vi "PictureControlIMAQReplacement.vi"() -> ()   [LabVIEW 2019]
uses:
  <vilib>/Utility/miscctls.llb/LVPoint32TypeDef.ctl
  <vilib>/Utility/miscctls.llb/LVPointTypeDef.ctl
  <vilib>/Utility/miscctls.llb/LVBoundsTypeDef.ctl
  <vilib>/Utility/error.llb/whitespace.ctl
  <userlib>/_OpenG.lib/array/array.llb/Reverse 2D Array (SGL)__ogtk.vi
  <vilib>/picture/picture.llb/Draw True-Color Pixmap.vi
  <vilib>/Dataflowg/G-Image/G-Image/Image Processing/Polymorphic VIs/Resize Image (Scale).vi
  Classes/Render/BigMAQ/BigMAQ.lvclass
  <vilib>/Dataflowg/G-Image/G-Image/G-Image.lvlib
panel:
  out "size(s) 3":i32
  out "size(s) 2":i32
  out "new picture":picture
  out "Array":picture[](array[picture])
  in  "Basename":string
  out "error out":errorcluster
  in  "error in (no error)":errorcluster
  out "Notes LUT":variant
  in  "Path":path
  out "NewVal":T1(ring)
  in  "Selection":T1(radio)
  out "Button":u16
  out "Draw Area Size":T2
  out "Origin":T3
  out "x-y":T4
  out "2D Picture":picture
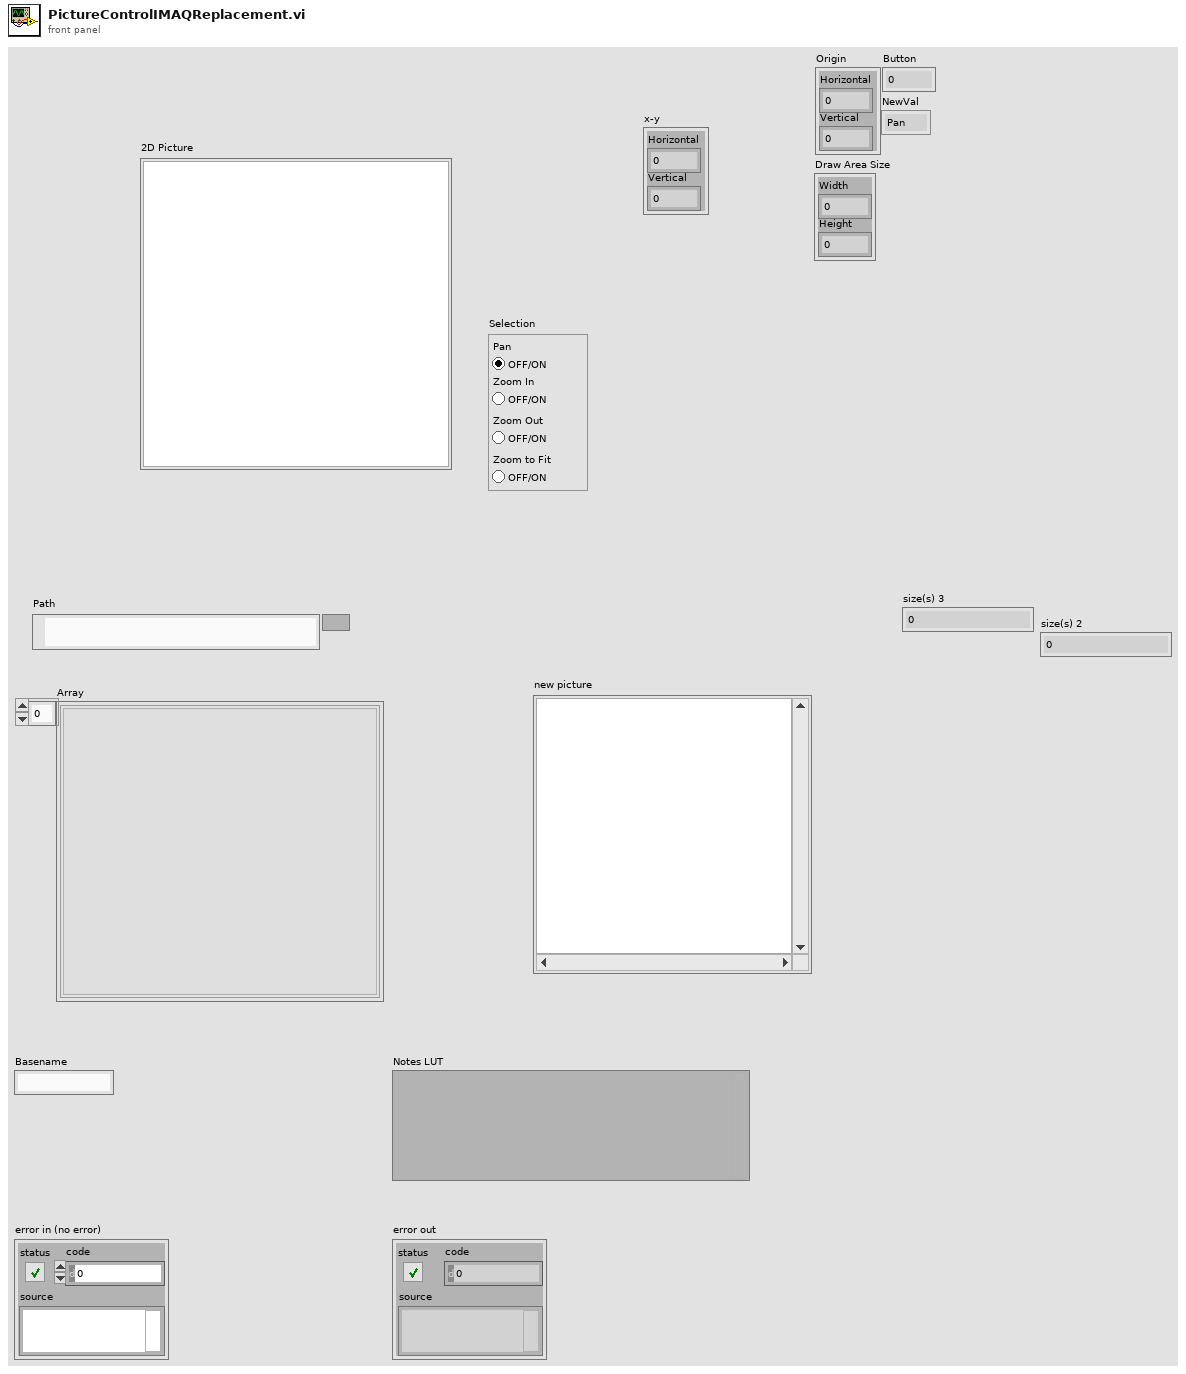
[diagram p1: front panel]
types:
  T1 = enum32{"Pan", "Zoom In", "Zoom Out", "Zoom to Fit"}
  T2 = typedef "LVBoundsTypeDef.ctl" = cluster{"Width":u32, "Height":u32}
  T3 = typedef "LVPointTypeDef.ctl" = cluster{"Horizontal":i16, "Vertical":i16}
  T4 = typedef "LVPoint32TypeDef.ctl" = cluster{"Horizontal":i32, "Vertical":i32}
  T5 = enum32{"Invalid", "Standard", "Closed", "Hidden", "Minimized", "Maximized"}
  T6 = enum32{"invalid app kind", "Development System", "Run Time System", "Student Edition", "Embedded LabVIEW", "Evaluation", "Custom"}
  T7 = enum16{"big-endian, network order", "native, host order", "little-endian"}
  T8 = cluster{"Core":cluster{"Current VI Reference":refnum<vi>, "Close Panel on Exit?":bool}, "Binary":string, "wfmSize":i32, "noteSize":i32, "nDim":i32[], "wData":sgl[], "Shaped wData":sgl[][][], "Notes":string, "Images":refnum<data-value>[]}
  T9 = cluster{"Current VI Reference":refnum<vi>, "Close Panel on Exit?":bool}
  T10 = typedef "whitespace.ctl" = u16
  T11 = typedef "imagedata.ctl" = cluster{"image type":i32, "image depth":i32, "image":u8[], "mask":u8[], "colors":u32[], "Rectangle":cluster{"left":i16, "top":i16, "right":i16, "bottom":i16}}
  T12 = cluster{"Core":cluster{"Current VI Reference":refnum<vi>, "Close Panel on Exit?":bool}, "MD Coords":T4, "MU Coords":T4, "MD":bool, "MD Origin":T4, "Selection":enum32{"Pan", "Zoom In", "Zoom Out", "Zoom to Fit"}}
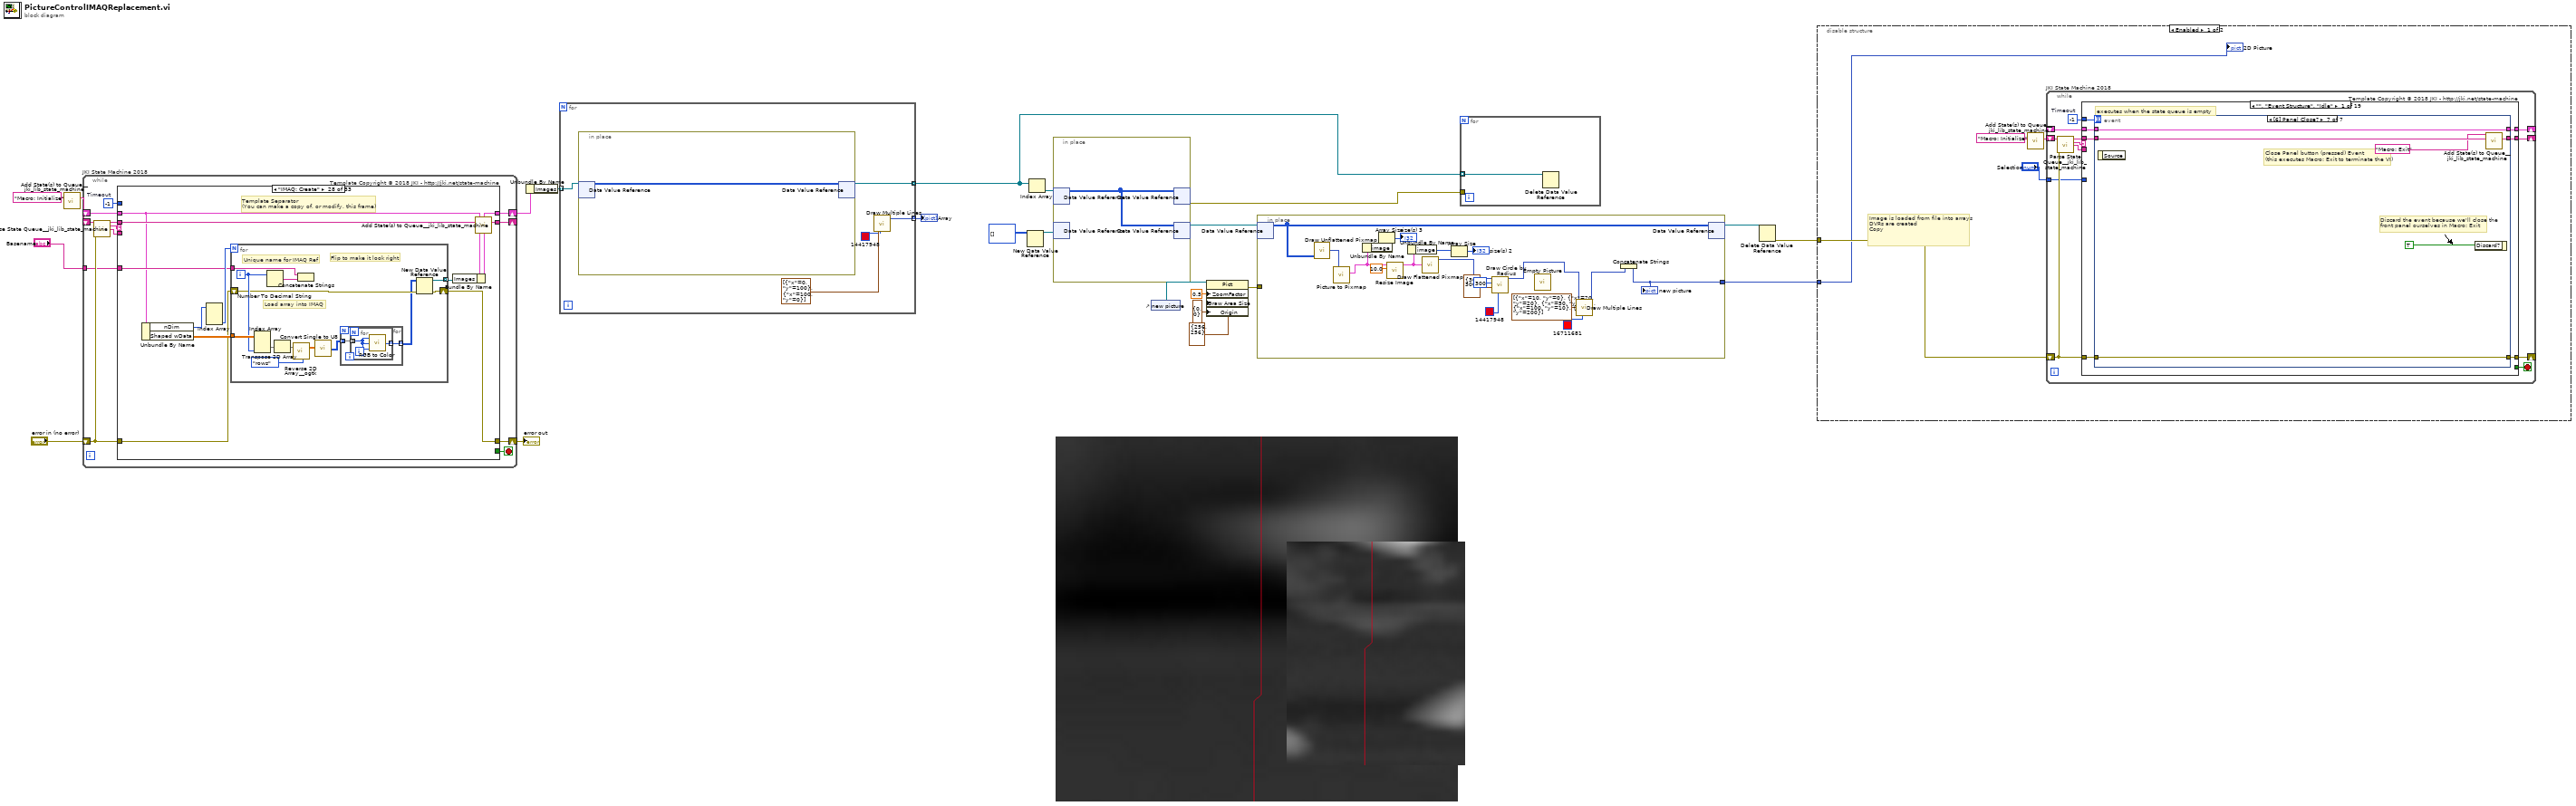
[diagram p0: block diagram]
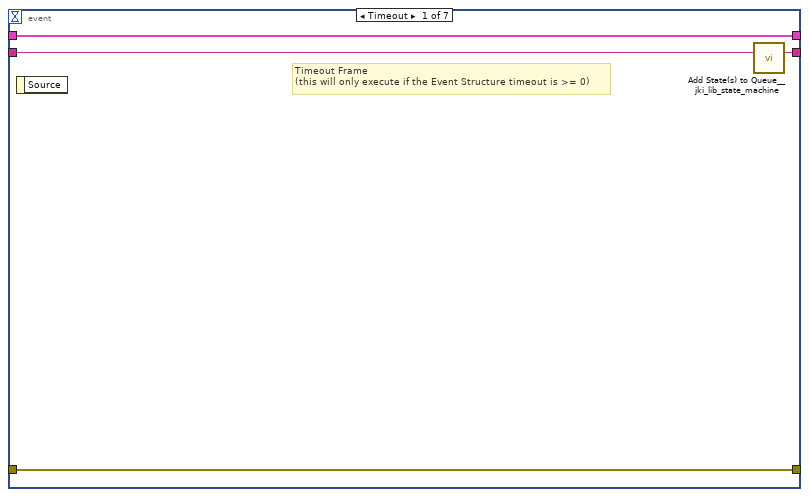
[diagram p2: hidden frame]
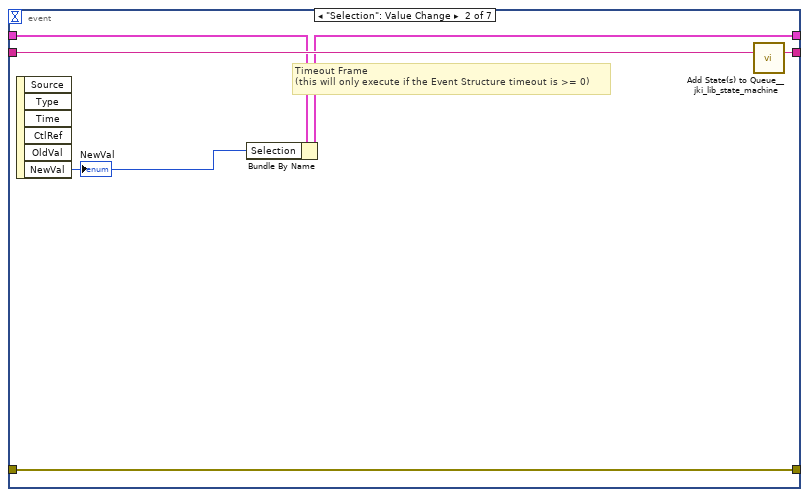
[diagram p3: hidden frame]
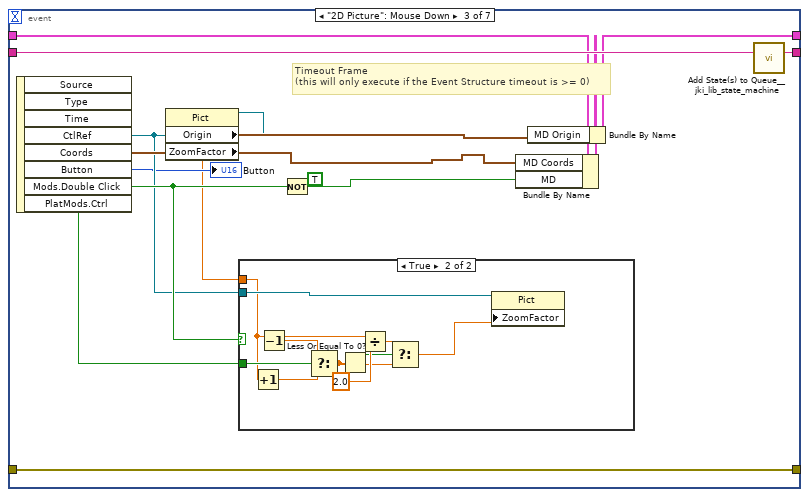
[diagram p4: hidden frame]
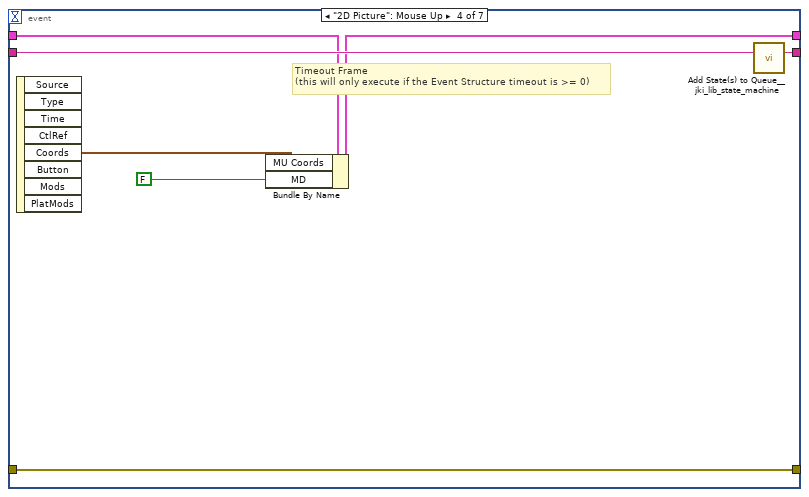
[diagram p6: hidden frame]
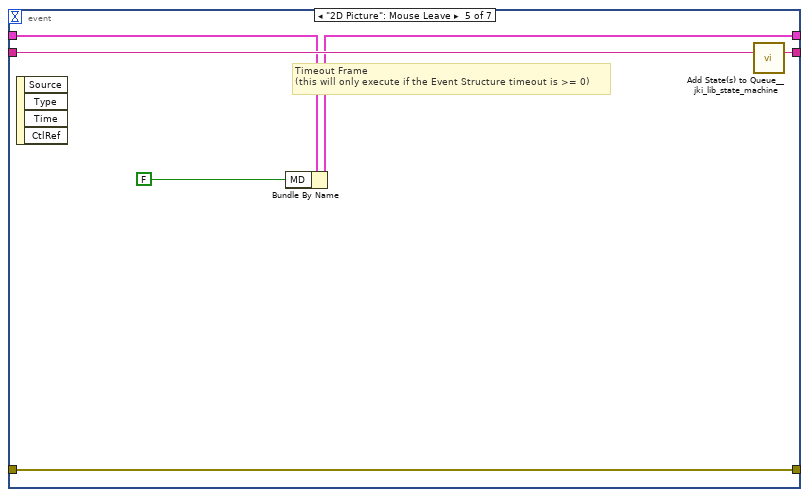
[diagram p7: hidden frame]
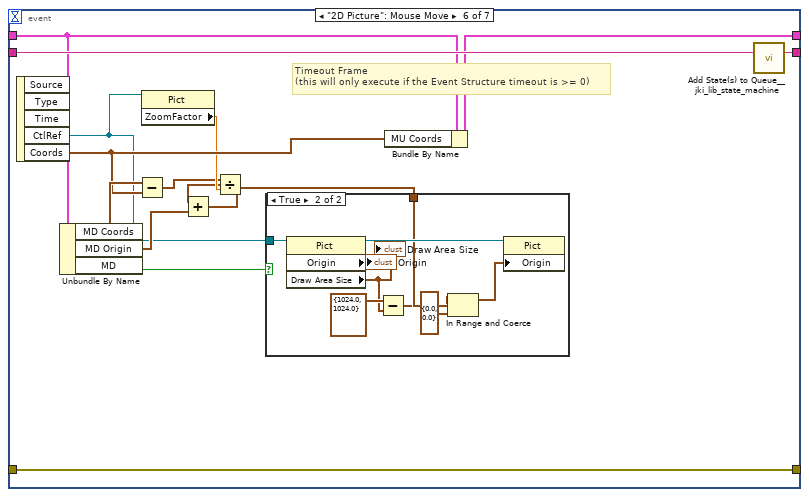
[diagram p8: hidden frame]
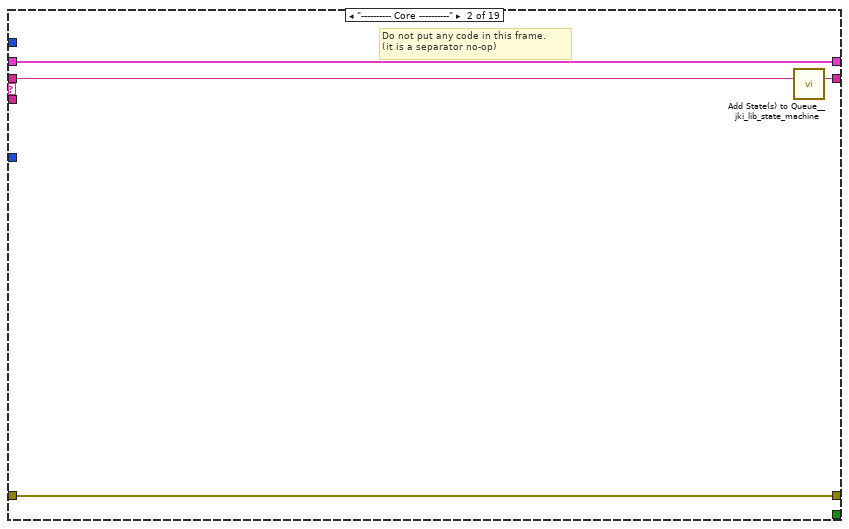
[diagram p10: hidden frame]
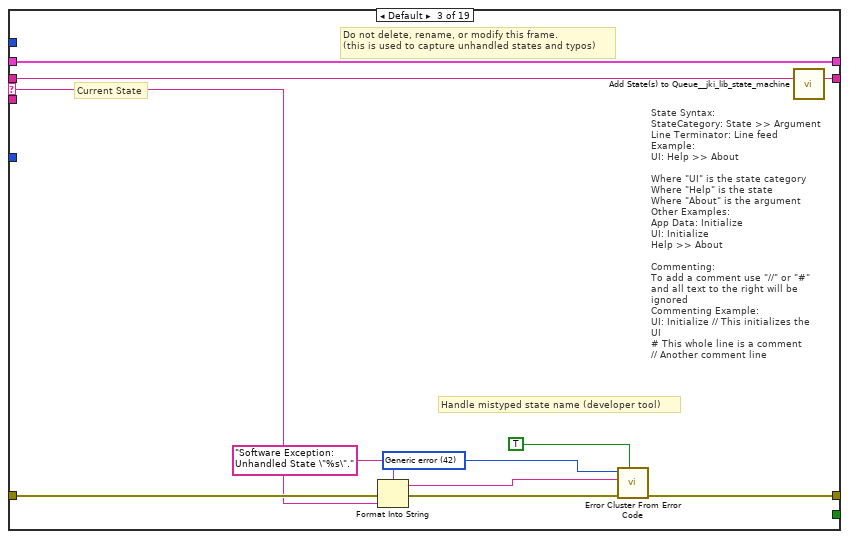
[diagram p11: hidden frame]
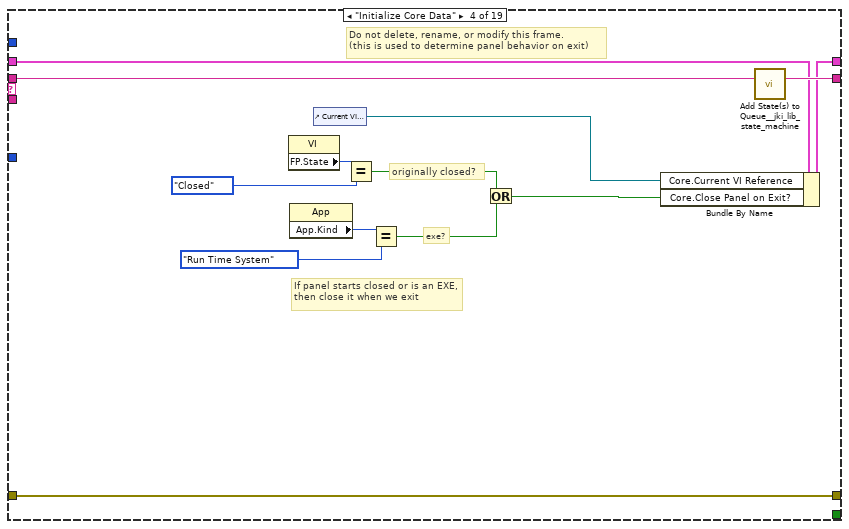
[diagram p12: hidden frame]
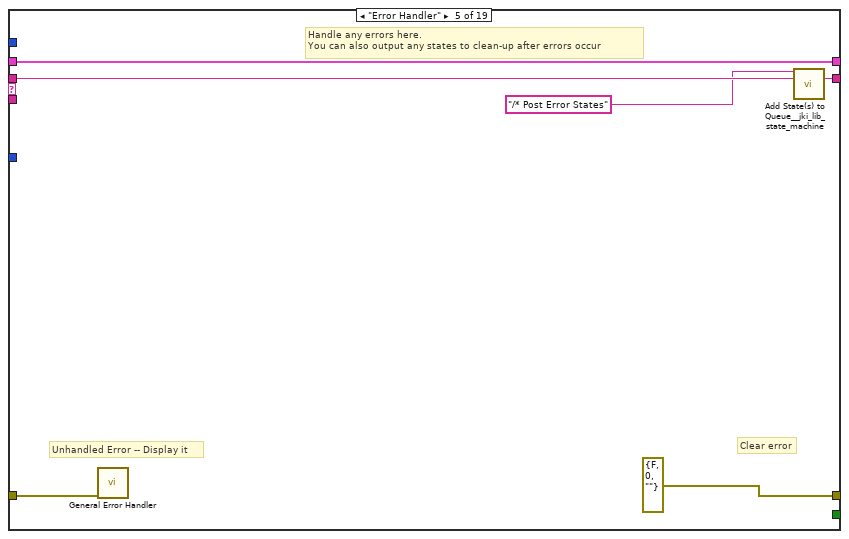
[diagram p13: hidden frame]
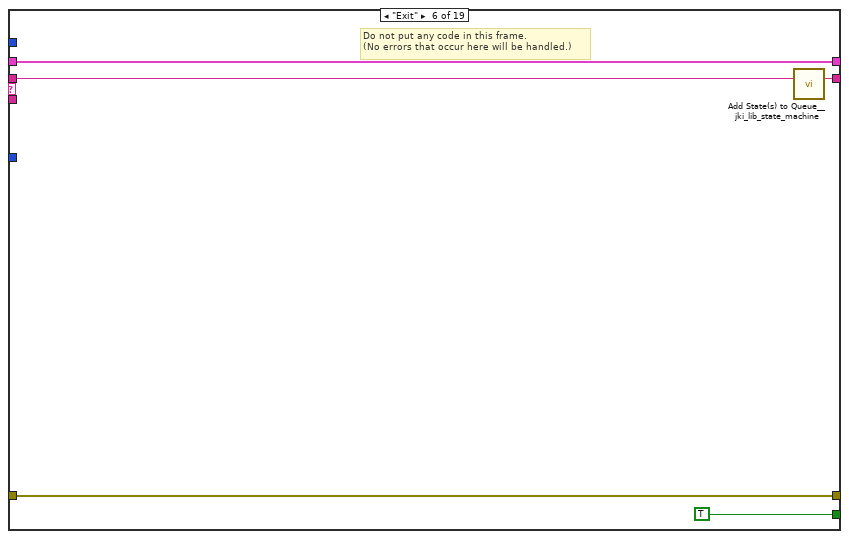
[diagram p14: hidden frame]
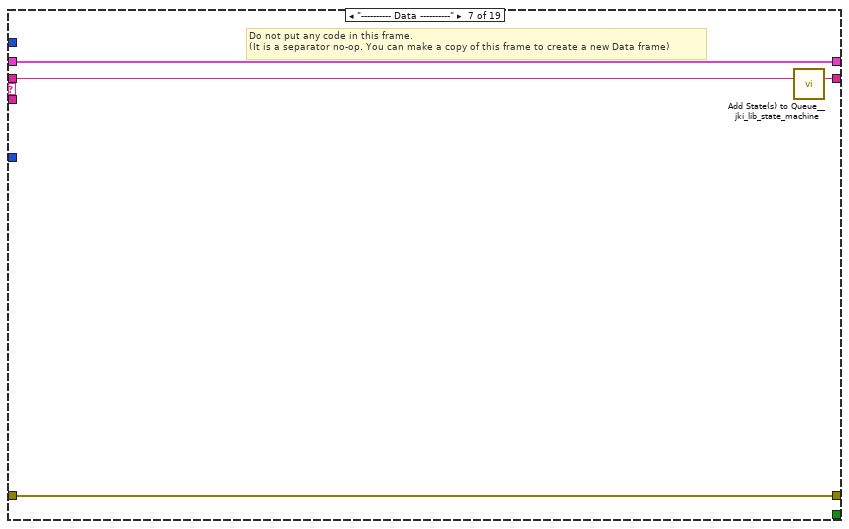
[diagram p15: hidden frame]
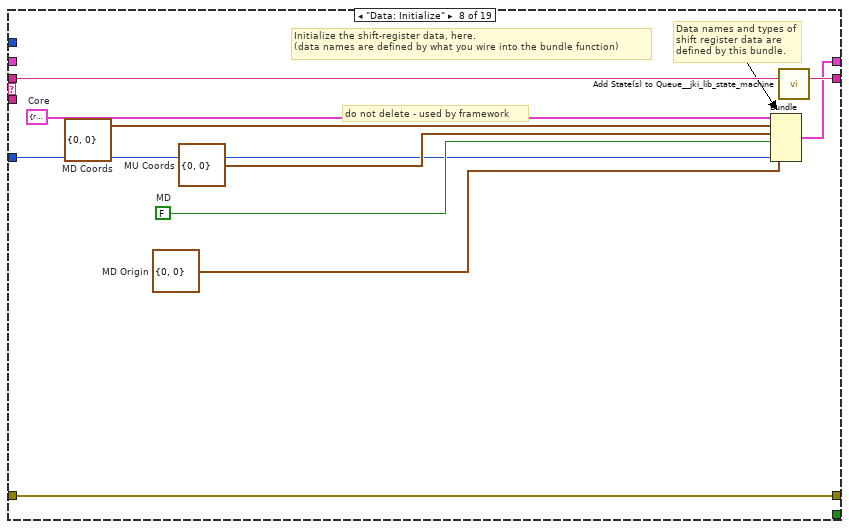
[diagram p16: hidden frame]
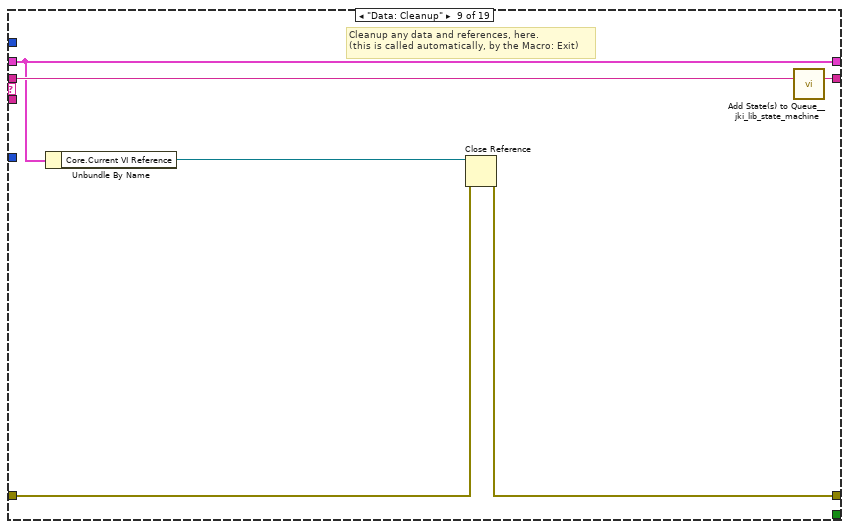
[diagram p17: hidden frame]
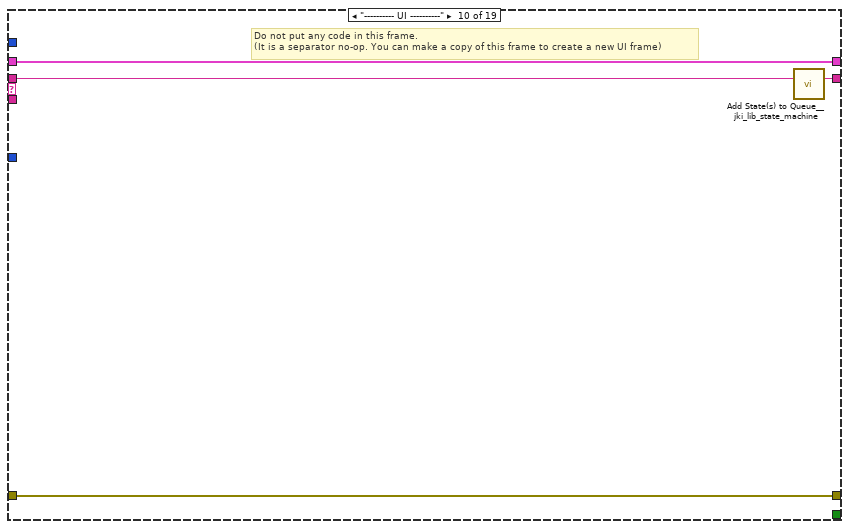
[diagram p18: hidden frame]
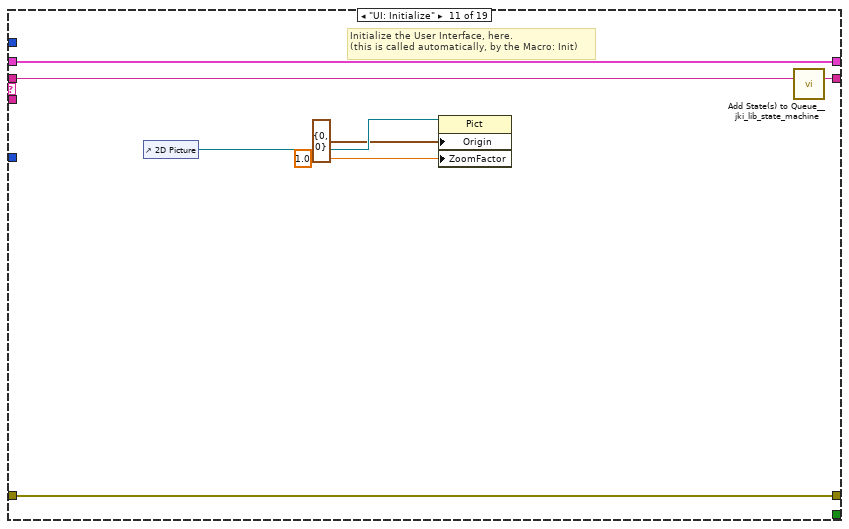
[diagram p19: hidden frame]
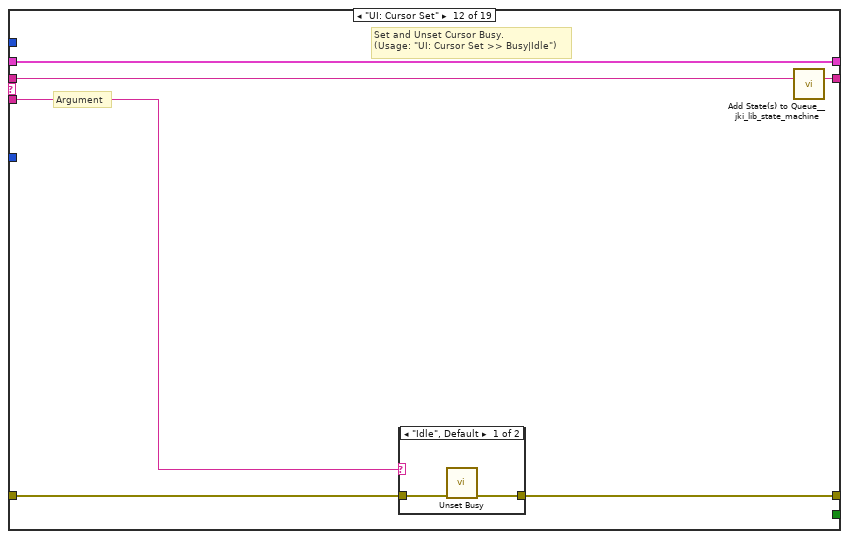
[diagram p20: hidden frame]
diagram:
  n1 = call <vilib>:"Add State(s) to Queue__jki_lib_state_machine.vi"("State(s) in (\"\")"="Macro: Initialize") -> ("States Out"=w22:string)  [unwired: 14 in]
  n2 = while "JKI State Machine 2018" {
    shift-right: [w27] -> w17
    shift-left: _ -> [w26]
    shift-right: [w30] -> w20
    shift-left: "error in (no error)" -> [w24]
    shift-right: [w29] -> _
    shift-left: w22 -> [w31]
    tunnel: "Basename" -> [w23]
    stop <- w28 stop-if-true
    w25 = -1  # Timeout
    # "Template Copyright © 2018 JKI - http://jki.net/state-machine"
    n3 = call <vilib>:"Parse State Queue__jki_lib_state_machine.vi"("State Queue"=w31, "Error In (no error)"=w24) -> ("Remaining States"=w33:string, "Current State"=w34:string, "Arguments"=w32:string)  [unwired: 11 in]
    n4 = case shown="\"IMAQ: Create\"" w34 {
      selector: w34 -> [_ _ w56 _ _ _ _ _ _ _ _ _ _ _ _ _ _ _ _ _ _ _ _ _ _ _ _ _ _ _ _ _ _]
      tunnel: w33 -> [w41 w55 w60 w79 w85 w90 w94 w107 w113 w117 w121 w127 w138 w207 w212 w217 w227 w231 w239 w243 w256 w269 w282 w303 w318 w354 w358 w369 w390 w400 w423 w427 w431]
      tunnel: w32 -> [_ _ _ _ _ _ _ _ _ _ _ w122 w132 _ _ _ _ _ _ _ _ _ _ _ _ _ _ _ _ _ _ _ _]
      tunnel: w26 -> [w39 w52 w58 w72 w82 w88 w91 _ w108 w114 w119 w125 w134 w204 w209 w214 w224 w228 w235 w240 w245 w258 w272 w293 w310 w345 w355 w360 w387 w398 w420 w424 w428]
      tunnel: [w38 w53 w62 w76 errorcluster {"status"=FALSE, "code"=0, "source"=""} ("error out") w87 w92 w104 w109 w115 w118 w123 w135 w205 w210 w215 w225 w229 w233 w241 w254 w267 w280 w284 w316 w352 w356 w363 w388 w392 w421 w425 w429] -> w30
      tunnel: w24 -> [w37 w53 w61 w76 w81 w87 w92 w104 w110 w115 w118 w124 w136 w205 w210 w215 w225 w229 w232 w241 w254 w267 w280 w285 w316 w352 w356 w364 w388 w391 w421 w425 w429]
      tunnel: [w40 w54 w59 w78 w84 w89 w93 w106 w112 w116 w120 w126 w137 w206 w211 w216 w226 w230 w238 w242 w255 w268 w281 w302 w317 w353 w357 w368 w389 w399 w422 w426 w430] -> w29
      tunnel: [_ _ _ _ _ TRUE _ _ _ _ _ _ _ _ _ _ _ _ _ _ _ _ _ _ _ _ _ _ _ _ _ _ _] -> w28
      tunnel: [w36 w52 w58 w77 w82 w88 w91 w105 w108 w114 w119 w125 w134 w204 w209 w214 w224 w228 w236 w240 w246 w259 w273 w294 w311 w346 w355 w361 w387 w398 w420 w424 w428] -> w27
      tunnel: w25 -> [w35 _ _ _ _ _ _ _ _ _ _ _ _ _ _ _ _ _ _ _ _ _ _ _ _ _ _ _ _ _ _ _ _]
      tunnel: w23 -> [_ _ _ _ _ _ _ _ _ _ _ _ _ _ _ _ _ _ _ _ _ _ _ _ _ _ _ w362 _ _ _ _ _]
      frame "", "Event Structure", "Idle" {
        # "executes when the state queue is empty"
        n5 = event shown="[1] Panel Close?" {
          selector: _ -> [_ _]
          dyn-events: _ -> [_ _]
          timeout: w35 -> [_ _]
          tunnel: w41 -> [w45 w51]
          tunnel: [w44 w50] -> w40
          tunnel: w39 -> [w42 w48]
          tunnel: [w43 w49] -> w38
          tunnel: w37 -> [w43 w49]
          tunnel: [w42 w48] -> w36
          event Timeout {
            n6 = event-data() -> ()  [unwired: 1 in, 1 out]
            n7 = call <vilib>:"Add State(s) to Queue__jki_lib_state_machine.vi"("State(s) in (\"\")"=w45) -> ("States Out"=w44:string)  [unwired: 14 in]
          }
          event Panel Close? {
            # "Discard the event because we'll close the front panel ourselves in Macro: Exit"
            # "Close Panel button (pressed) Event\n(this executes Macro: Exit to terminate the VI)"
            n8 = event-data() -> ()  [unwired: 1 in, 1 out]
            n9 = event-data ("Event Filter Node")("Discard?"=TRUE) -> ()  [unwired: 1 in, 1 out]
            n10 = call <vilib>:"Add State(s) to Queue__jki_lib_state_machine.vi"("State(s) in Front (\"\")"="Macro: Exit", "State(s) in (\"\")"=w51) -> ("States Out"=w50:string)  [unwired: 13 in]
          }
        }
      }
      frame "---------- Core ----------" {
        # "Do not put any code in this frame.\n(it is a separator no-op)"
        n11 = call <vilib>:"Add State(s) to Queue__jki_lib_state_machine.vi"("State(s) in (\"\")"=w55) -> ("States Out"=w54:string)  [unwired: 14 in]
      }
      frame Default {
        w65 = 42 items=["No error", "Argument error", "Memory is full", "Out of zone", "End of file", "File already open", "Generic file I/O error", "File not found", "File permission error", "Disk is full", "Duplicate path", "Too many files open", "System feature not enabled", "Resource file not found", "Cannot add resource", "Resource not found", "Image not found", "Image memory error", "Pen does not exist", "Config type invalid", "Config token not found", "Config parse error", "Config memory error", "Bad external code format", "Bad external code offset", "External code not present", "Null window", "Destroy window error", "Null menu", "Print aborted", "Bad print record", "Print driver error", "Windows error during printing", "Memory error during printing", "Print dialog error", "Generic print error", "Invalid device refnum", "Device not found", "Device parameter error", "Device unit error", "Cannot open device", "Device call aborted", "Generic error", "Cancelled by user", "Object ID too low", "Object ID too high", "Object not in heap", "Unknown heap", "Unknown object (invalid DefProc)", "Unknown object (DefProc not in table)", "Message out of range", "Invalid (null) method", "Unknown message", "Manager call not supported", "Bad address", "Network operation in progress", "Network operation timed out", "Connection is busy", "Network attribute not supported", "Network error", "Address in use", "System out of memory", "Connection aborted", "Connection refused", "Not connected", "Already connected", "Connection closed", "Initialization error (interapplication manager)", "Bad occurrence", "Wait on unbound occurrence handler", "Occurrence queue overflow", "Datalog type conflict", "Unused", "Unrecognized type (interapplication manager)", "Memory corrupt", "Failed to make temporary DLL", "Old CIN version", "Drag socket not found", "Failed to load drop-object", "Failed to register OLE object", "Failed to release OLE object", "Format specifier type mismatch", "Unknown format specifier", "Too few format specifiers", "Too many format specifiers", "Scan failed", "Newer CIN version", "Error converting to variant", "Runtime menu error", "Password tampered", "Variant attribute not found", "Incompatible variant data type", "Event data is not available", "Event Store is not present", "Occurrence is not found", "Event Queue is not created", "Event info is not available", "Refnum passed is NULL", "Error retrieving Class GUID", "Error retrieving CoClass GUID", "Error retrieving TypeLib GUID.", "Bad built application magic bytes.", "Specific driver is different from the specific driver associated with the Logical Name.", "There is no session opened to the class driver.", "Max Error", "MAX - Error with config objects", "MAX - Error loading configuration", "MAX - Group not supported"]
        # "Current State"
        # "Do not delete, rename, or modify this frame.\n(this is used to capture unhandled states and typos)"
        # "Handle mistyped state name (developer tool)"
        n12 = Format Into String(format string="Software Exception: Unhandled State \"%s\"." ("message"), error in=w61, w56) -> (resulting string=w64:string, error out=w63:errorcluster)  [unwired: 1 in]
        n13 = call <vilib>:"Error Cluster From Error Code.vi"("show call chain? (False)"=TRUE, "error in (no error)"=w63, "error message (\"\")"=w64, "error code (0)"=w65) -> ("error out"=w62:errorcluster)  [unwired: 5 in]
        n14 = call <vilib>:"Add State(s) to Queue__jki_lib_state_machine.vi"("State(s) in (\"\")"=w60) -> ("States Out"=w59:string)  [unwired: 14 in]
      }
      frame "Initialize Core Data" {
        # "Do not delete, rename, or modify this frame.\n(this is used to determine panel behavior on exit)"
        # "originally closed?"
        # "exe?"
        # "If panel starts closed or is an EXE, then close it when we exit"
        n15 = property on="Property Node" class="VI"() -> ("FP.State"=w69:T5)  [unwired: 2 in, 2 out]
        n16 = property on="Property Node" class="App"() -> ("App.Kind"=w75:T6)  [unwired: 2 in, 2 out]
        n17 = control-ref of="Current VI Reference"() -> (w70:refnum<vi>)
        n18 = Equal?(x=w69, y=T5."Closed" ("Front Panel Window:State")) -> (x = y?=w67:bool)
        n19 = Equal?(x=w75, y=T6."Run Time System" ("Application:Kind")) -> (x = y?=w73:bool)
        n20 = Or(x=w67, y=w73) -> (x .or. y?=w71:bool)
        n21 = Bundle By Name(cluster=w72, "Core.Current VI Reference"=w70, "Core.Close Panel on Exit?"=w71) -> (w77:T8)
        n22 = call <vilib>:"Add State(s) to Queue__jki_lib_state_machine.vi"("State(s) in (\"\")"=w79) -> ("States Out"=w78:string)  [unwired: 14 in]
      }
      frame "Error Handler" {
        # "Unhandled Error -- Display it"
        # "Handle any errors here.\nYou can also output any states to clean-up after errors occur"
        # "Clear error"
        n23 = call <vilib>:"General Error Handler.vi"("error in (no error)"=w81) -> ()  [unwired: 10 in, 5 out]
        n24 = call <vilib>:"Add State(s) to Queue__jki_lib_state_machine.vi"("State(s) in Front (\"\")"="/* Post Error States", "State(s) in (\"\")"=w85) -> ("States Out"=w84:string)  [unwired: 13 in]
      }
      frame "Exit" {
        # "Do not put any code in this frame.\n(No errors that occur here will be handled.)"
        n25 = call <vilib>:"Add State(s) to Queue__jki_lib_state_machine.vi"("State(s) in (\"\")"=w90) -> ("States Out"=w89:string)  [unwired: 14 in]
      }
      frame "---------- Data ----------" {
        # "Do not put any code in this frame.\n(It is a separator no-op. You can make a copy of this frame to create a new Data frame)"
        n26 = call <vilib>:"Add State(s) to Queue__jki_lib_state_machine.vi"("State(s) in (\"\")"=w94) -> ("States Out"=w93:string)  [unwired: 14 in]
      }
      frame "Data: Initialize" {
        (unwired) refnum<data-value> refnum  # Image Data
        w95 = refnum<data-value>[] []  # Images
        w96 = ""  # Notes
        w97 = sgl[][][] []  # Shaped wData
        w98 = sgl[] []  # wData
        w99 = i32[] []  # nDim
        w100 = 0  # noteSize
        w101 = 0  # wfmSize
        w102 = T9 {"Current VI Reference"=refnum, "Close Panel on Exit?"=FALSE}  # Core
        w103 = ""  # Binary
        # "do not delete - used by framework"
        # "Add new data here."
        # "Data names and types of shift register data are defined by this bundle."
        # "Initialize the shift-register data, here.\n(data names are defined by what you wire into the bundle function)"
        n27 = Bundle("Core"=w102, "Binary"=w103, "wfmSize"=w101, "noteSize"=w100, "nDim"=w99, "wData"=w98, "Shaped wData"=w97, "Notes"=w96, "Images"=w95) -> (w105:T8)  [unwired: 1 in]
        n28 = call <vilib>:"Add State(s) to Queue__jki_lib_state_machine.vi"("State(s) in (\"\")"=w107) -> ("States Out"=w106:string)  [unwired: 14 in]
      }
      frame "Data: Cleanup" {
        # "Cleanup any data and references, here.\n(this is called automatically, by the Macro: Exit)"
        n29 = Unbundle By Name(w108) -> ("Core.Current VI Reference"=w111:refnum<vi>)
        n30 = Close Reference(reference=w111, error in (no error)=w110) -> (error out=w109:errorcluster)
        n31 = call <vilib>:"Add State(s) to Queue__jki_lib_state_machine.vi"("State(s) in (\"\")"=w113) -> ("States Out"=w112:string)  [unwired: 14 in]
      }
      frame "---------- UI ----------" {
        # "Do not put any code in this frame.\n(It is a separator no-op. You can make a copy of this frame to create a new UI frame)"
        n32 = call <vilib>:"Add State(s) to Queue__jki_lib_state_machine.vi"("State(s) in (\"\")"=w117) -> ("States Out"=w116:string)  [unwired: 14 in]
      }
      frame "UI: Initialize" {
        # "Initialize the User Interface, here.\n(this is called automatically, by the Macro: Init)"
        n33 = call <vilib>:"Add State(s) to Queue__jki_lib_state_machine.vi"("State(s) in (\"\")"=w121) -> ("States Out"=w120:string)  [unwired: 14 in]
      }
      frame "UI: Cursor Set" {
        # "Argument"
        # "Set and Unset Cursor Busy.\n(Usage: \"UI: Cursor Set >> Busy|Idle\")"
        n34 = case shown="\"Busy\"" w122 {
          tunnel: w124 -> [w129 w131]
          tunnel: [w128 w130] -> w123
          frame "Idle", Default {
            n35 = call <vilib>:"Unset Busy.vi"("error in (no error)"=w129) -> ("error out"=w128:errorcluster)  [unwired: 10 in]
          }
          frame "Busy" {
            n36 = call <vilib>:"Set Busy.vi"("error in (no error)"=w131) -> ("error out"=w130:errorcluster)  [unwired: 9 in, 1 out]
          }
        }
        n37 = call <vilib>:"Add State(s) to Queue__jki_lib_state_machine.vi"("State(s) in (\"\")"=w127) -> ("States Out"=w126:string)  [unwired: 14 in]
      }
      frame "UI: Front Panel State" {
        # "Argument"
        # "Set Front Panel Open or Closed\n(Usage: \"UI: Front Panel State >> Open|Close\")"
        n38 = Unbundle By Name(w134) -> ("Core.Current VI Reference"=w133:refnum<vi>)
        n39 = case shown="\"Minimize\", \"Minimized\"" w132 {
          tunnel: w136 -> [w144 w159 w170 w183 w196]
          tunnel: [w146 w160 w172 w185 w198] -> w135
          tunnel: w133 -> [w145 w157 w171 w184 w197]
          frame "Open", "Standard", Default {
            w139 = T5."Standard" ("State")
            n40 = property on="Property Node" class="VI"(reference=w145, error in=w144) -> (reference out=w142:refnum<vi>, error out=w143:errorcluster, "FP.State"=w141:T5)
            n41 = Not Equal?(x=w141, y=w139) -> (x != y?=w140:bool)
            n42 = case shown="True" w140 {
              tunnel: [w150 w152] -> w146
              tunnel: w143 -> [w149 w152]
              tunnel: w142 -> [w148 _]
              tunnel: w139 -> [w147 _]
              frame True {
                n43 = invoke on="Invoke Node" class="VI" method="FP.Open"(reference=w148, error in=w149, "Activate"=TRUE, "State"=w147) -> (error out=w150:errorcluster)  [unwired: 1 in, 4 out]
              }
              frame False {
              }
            }
          }
          frame "Close", "Closed" {
            n44 = property on="Property Node" class="VI"(reference=w157, error in=w159) -> (reference out=w156:refnum<vi>, error out=w158:errorcluster, "FP.State"=w154:T5)
            n45 = Not Equal?(x=w154, y=T5."Closed" ("Front Panel Window:State")) -> (x != y?=w153:bool)
            n46 = case shown="True" w153 {
              tunnel: [w161 w164] -> w160
              tunnel: w158 -> [w161 w163]
              tunnel: w156 -> [_ w162]
              frame False {
              }
              frame True {
                n47 = invoke on="Invoke Node" class="VI" method="FP.Close"(reference=w162, error in=w163) -> (error out=w164:errorcluster)  [unwired: 1 in, 2 out]
              }
            }
          }
          frame "Hidden", "Hide" {
            w165 = T5."Hidden" ("State")
            n48 = property on="Property Node" class="VI"(reference=w171, error in=w170) -> (reference out=w168:refnum<vi>, error out=w169:errorcluster, "FP.State"=w167:T5)
            n49 = Not Equal?(x=w167, y=w165) -> (x != y?=w166:bool)
            n50 = case shown="True" w166 {
              tunnel: [w176 w177] -> w172
              tunnel: w169 -> [w175 w177]
              tunnel: w168 -> [w174 _]
              tunnel: w165 -> [w173 _]
              frame True {
                n51 = invoke on="Invoke Node" class="VI" method="FP.Open"(reference=w174, error in=w175, "State"=w173) -> (error out=w176:errorcluster)  [unwired: 2 in, 4 out]
              }
              frame False {
              }
            }
          }
          frame "Minimize", "Minimized" {
            w178 = T5."Minimized" ("State")
            n52 = property on="Property Node" class="VI"(reference=w184, error in=w183) -> (reference out=w181:refnum<vi>, error out=w182:errorcluster, "FP.State"=w180:T5)
            n53 = Not Equal?(x=w180, y=w178) -> (x != y?=w179:bool)
            n54 = case shown="True" w179 {
              tunnel: [w189 w190] -> w185
              tunnel: w182 -> [w188 w190]
              tunnel: w181 -> [w187 _]
              tunnel: w178 -> [w186 _]
              frame True {
                n55 = invoke on="Invoke Node" class="VI" method="FP.Open"(reference=w187, error in=w188, "State"=w186) -> (error out=w189:errorcluster)  [unwired: 2 in, 4 out]
              }
              frame False {
              }
            }
          }
          frame "Maximize", "Maximized" {
            w191 = T5."Maximized" ("State")
            n56 = property on="Property Node" class="VI"(reference=w197, error in=w196) -> (reference out=w194:refnum<vi>, error out=w195:errorcluster, "FP.State"=w193:T5)
            n57 = Not Equal?(x=w193, y=w191) -> (x != y?=w192:bool)
            n58 = case shown="True" w192 {
              tunnel: [w202 w203] -> w198
              tunnel: w195 -> [w201 w203]
              tunnel: w194 -> [w200 _]
              tunnel: w191 -> [w199 _]
              frame True {
                n59 = invoke on="Invoke Node" class="VI" method="FP.Open"(reference=w200, error in=w201, "State"=w199) -> (error out=w202:errorcluster)  [unwired: 2 in, 4 out]
              }
              frame False {
              }
            }
          }
        }
        n60 = call <vilib>:"Add State(s) to Queue__jki_lib_state_machine.vi"("State(s) in (\"\")"=w138) -> ("States Out"=w137:string)  [unwired: 14 in]
      }
      frame "---------- Macro ----------" {
        # "Backups in case Directory State gets deleted on accident since those are never called"
        # "Length|Index|typedef struct BinHeader5 {\n     2|    0|\tshort version;\t\t\t\t\t\t          // Version number for backwards compatibility.\n     2|    2|\tshort checksum;\t\t\t\t\t\t         // Checksum over this header and the wave header.\n     4|    4|\tlong wfmSize;\t\t\t\t\t\t           // The size of the WaveHeader5 data structure plus the wave data.\n     4|    8|\tlong formulaSize;\t\t\t\t\t        // The size of the dependency formula, if any.\n     4|   12|\tlong noteSize;\t\t\t\t\t\t          // The size of the note text.\n     4|   16|\tlong dataEUnitsSize;\t\t\t\t      // The size of optional extended data units.\n    16|   20|\tlong dimEUnitsSize[MAXDIMS];\t\t// The size of optional extended dimension units.\n    16|   36|\tlong dimLabelsSize[MAXDIMS];\t\t// The size of optional dimension labels.\n     4|   52|\tlong sIndicesSize;\t\t\t\t\t       // The size of string indicies if this is a text wave.\n     4|   56|\tlong optionsSize1;\t\t\t\t\t       // Reserved. Write zero. Ignore on read.\n     4|   60|\tlong optionsSize2;\t\t\t\t\t       // Reserved. Write zero. Ignore on read.\n      |   64|} BinHeader5;"
        # "Length|Index|struct WaveHeader5 {\n     4|   64|\tstruct WaveHeader5 **next;\t\t\t  // link to next wave in linked list.\n     4|   68|\tunsigned long creationDate;\t\t \t// DateTime of creation.\n     4|   72|\tunsigned long modDate;\t\t\t\t     // DateTime of last modification.\n     4|   76|\tlong npnts;\t\t\t\t\t\t\t             // Total number of points (multiply dimensions up to first zero).\n     2|   80|\tshort type;\t\t\t\t\t\t\t             // See types (e.g. NT_FP64) above. Zero for text waves.\n     2|   82|\tshort dLock;\t\t\t\t\t\t             // Reserved. Write zero. Ignore on read.\n     6|   84|\tchar whpad1[6];\t\t\t\t\t\t          // Reserved. Write zero. Ignore on read.\n     2|   90|\tshort whVersion;\t\t\t\t\t          // Write 1. Ignore on read.\n    32|   92|\tchar bname[MAX_WAVE_NAME5+1];\t\t// Name of wave plus trailing null.\n     4|  124|\tlong whpad2;\t\t\t\t\t\t             // Reserved. Write zero. Ignore on read.\n     4|  128|\tstruct DataFolder **dFolder;\t\t // Used in memory only. Write zero. Ignore on read.\n      |     |\t// Dimensioning info. [0] == rows, [1] == cols etc\n    16|  132|\tlong nDim[MAXDIMS];\t\t\t\t\t       // Number of of items in a dimension -- 0 means no data.\n    32|  148|\tdouble sfA[MAXDIMS];\t\t\t\t       // Index value for element e of dimension d = sfA[d]*e + sfB[d].\n    32|  180|\tdouble sfB[MAXDIMS];\n      |     |\t// SI units\n     4|  212|\tchar dataUnits[MAX_UNIT_CHARS+1];\t\t\t      // Natural data units go here - null if none.\n    16|  216|\tchar dimUnits[MAXDIMS][MAX_UNIT_CHARS+1];\t// Natural dimension units go here - null if none.\n     2|  232|\tshort fsValid;\t\t\t\t\t\t                      // TRUE if full scale values have meaning.\n     2|  234|\tshort whpad3;\t\t\t\t\t\t                       // Reserved. Write zero. Ignore on read.\n    16|  236|\tdouble topFullScale,botFullScale;\t        // The max and max full scale value for wave.\n     4|  252|\tHandle dataEUnits;\t\t\t\t\t                   // Used in memory only. Write zero. Ignore on read.\n    16|  256|\tHandle dimEUnits[MAXDIMS];\t\t\t             // Used in memory only. Write zero. Ignore on read.\n    16|  272|\tHandle dimLabels[MAXDIMS];\t\t\t             // Used in memory only. Write zero. Ignore on read.\n     4|  288|\tHandle waveNoteH;\t\t\t\t\t                    // Used in memory only. Write zero. Ignore on read.\n    64|  292|\tlong whUnused[16];\t\t\t\t\t                   // Reserved. Write zero. Ignore on read.\n      |     |\t// The following stuff is considered private to Igor.\n     2|  356|\tshort aModified;\t\t\t\t\t                     // Used in memory only. Write zero. Ignore on read.\n     2|  358|\tshort wModified;\t\t\t\t\t                     // Used in memory only. Write zero. Ignore on read.\n     2|  360|\tshort swModified;\t\t\t\t\t                    // Used in memory only. Write zero. Ignore on read.\n     1|  362|\tchar useBits;\t\t\t\t\t\t                       // Used in memory only. Write zero. Ignore on read.\n     1|  363|\tchar kindBits;\t\t\t\t\t\t                      // Reserved. Write zero. Ignore on read.\n     4|  364|\tvoid **formula;\t\t\t\t\t\t                     // Used in memory only. Write zero. Ignore on read.\n     4|  368|\tlong depID;\t\t\t\t\t\t\t                        // Used in memory only. Write zero. Ignore on read.\n     2|  372|\tshort whpad4;\t\t\t\t\t\t                       // Reserved. Write zero. Ignore on read.\n     2|  374|\tshort srcFldr;\t\t\t\t\t\t                      // Used in memory only. Write zero. Ignore on read.\n     4|  376|\tHandle fileName;\t\t\t\t\t                     // Used in memory only. Write zero. Ignore on read.\n     4|  380|\tlong **sIndices;\t\t\t\t\t                     // Used in memory only. Write zero. Ignore on read.\n     4|  384|\tfloat wData[1];\t\t\t\t\t\t                     // The start of the array of data. Must be 64 bit aligned.\n      |  388|};"
        # "Do not put any code in this frame.\n(It is a separator no-op. You can make a copy of this frame to create a new Macro frame)"
        n61 = call <vilib>:"Add State(s) to Queue__jki_lib_state_machine.vi"("State(s) in (\"\")"=w207) -> ("States Out"=w206:string)  [unwired: 14 in]
      }
      frame "Macro: Initialize" {
        # "Initialization Macro\n(This is called once, when the VI starts)"
        n62 = call <vilib>:"Add State(s) to Queue__jki_lib_state_machine.vi"("State(s) in Front (\"\")"="Data: Initialize\nInitialize Core Data\n//UI: Initialize\n//UI: Front Panel State >> Open\n\nMacro: Parse IBW\n\nMacro: Exit", "State(s) in (\"\")"=w212) -> ("States Out"=w211:string)  [unwired: 13 in]
      }
      frame "Macro: Parse IBW" {
        # "Parse IBW Macro\n(This is called once, when the VI starts)"
        n63 = call <vilib>:"Add State(s) to Queue__jki_lib_state_machine.vi"("State(s) in Front (\"\")"="File: Read\nParse: wfmSize\nParse: noteSize\nParse: nDim\nParse: wData\nParse: Shape wData\nParse: Notes\nIMAQ: Create\nNotes: Create LUT", "State(s) in (\"\")"=w217) -> ("States Out"=w216:string)  [unwired: 13 in]
      }
      frame "Macro: Exit" {
        # "Exit Macro\n(This is called once, when the VI exits)"
        n64 = Unbundle By Name(w224) -> ("Core.Close Panel on Exit?"=w223:bool)
        n65 = Select(t="UI: Front Panel State >> Close", s=w223, f="" ("Empty String Constant")) -> (s? t:f=w220:string)
        n66 = call <vilib>:"Add State(s) to Queue__jki_lib_state_machine.vi"("State(s) in (\"\")"=w220, "State(s) at Back (\"\")"="Data: Cleanup\nExit") -> ("States Out"=w218:string)  [unwired: 13 in]
        n67 = call <vilib>:"Add State(s) to Queue__jki_lib_state_machine.vi"("State(s) in Front (\"\")"=w218, "State(s) in (\"\")"=w227) -> ("States Out"=w226:string)  [unwired: 13 in]
      }
      frame "---------- File ----------" {
        # "Template Separator\n(You can make a copy of, or modify, this frame)"
        n68 = call <vilib>:"Add State(s) to Queue__jki_lib_state_machine.vi"("State(s) in (\"\")"=w231) -> ("States Out"=w230:string)  [unwired: 14 in]
      }
      frame "File: Read" {
        # "Ensure that Convert EOL? is set to False."
        # "File: Read\n(read characters from file)"
        n69 = Read from Text File(file (use dialog)="Path", error in=w232) -> (text=w234:string, error out=w233:errorcluster)  [unwired: 2 in, 2 out]
        n70 = Bundle By Name(cluster=w235, "Binary"=w234) -> (w236:T8)
        n71 = call <vilib>:"Add State(s) to Queue__jki_lib_state_machine.vi"("State(s) in (\"\")"=w239) -> ("States Out"=w238:string)  [unwired: 14 in]
      }
      frame "---------- Parse ----------" {
        # "Template Separator\n(You can make a copy of, or modify, this frame)"
        n72 = call <vilib>:"Add State(s) to Queue__jki_lib_state_machine.vi"("State(s) in (\"\")"=w243) -> ("States Out"=w242:string)  [unwired: 14 in]
      }
      frame "Parse: wfmSize" {
        # "From Big Endian to Little Endian"
        # "Convert to integer"
        # "Location: See Directory"
        # "Parse: wfmSize\n(*)"
        n73 = Unbundle By Name(w245) -> ("Binary"=w253:string)
        n74 = String Subset(string=w253, offset (0)=4, length (rest)=4 ("length (rest)")) -> (substring=w250:string)
        n75 = Type Cast(type=0, x=w250) -> (*(type *) &x=w248:i32)
        n76 = Swap Bytes(anything=w248) -> (byte swapped=w249:i32)
        n77 = Swap Words(1:w249) -> (0:w244:i32)
        n78 = Bundle By Name(cluster=w245, "wfmSize"=w244) -> (w246:T8)
        n79 = call <vilib>:"Add State(s) to Queue__jki_lib_state_machine.vi"("State(s) in (\"\")"=w256) -> ("States Out"=w255:string)  [unwired: 14 in]
      }
      frame "Parse: noteSize" {
        # "From Big Endian to Little Endian"
        # "Convert to integer"
        # "Location: See Directory"
        # "Parse: noteSize\n(*)"
        n80 = Unbundle By Name(w258) -> ("Binary"=w266:string)
        n81 = String Subset(string=w266, offset (0)=12, length (rest)=4 ("length (rest)")) -> (substring=w263:string)
        n82 = Type Cast(type=0, x=w263) -> (*(type *) &x=w261:i32)
        n83 = Swap Bytes(anything=w261) -> (byte swapped=w262:i32)
        n84 = Swap Words(1:w262) -> (0:w257:i32)
        n85 = Bundle By Name(cluster=w258, "noteSize"=w257) -> (w259:T8)
        n86 = call <vilib>:"Add State(s) to Queue__jki_lib_state_machine.vi"("State(s) in (\"\")"=w269) -> ("States Out"=w268:string)  [unwired: 14 in]
      }
      frame "Parse: nDim" {
        # "From Big Endian to Little Endian"
        # "Convert to integer"
        # "Location: See Directory"
        # "Parse: nDim\n(*)"
        n87 = Unbundle By Name(w272) -> ("Binary"=w274:string)
        n88 = String Subset(string=w274, offset (0)=132, length (rest)=16 ("length (rest)")) -> (substring=w279:string)
        n89 = Type Cast(type=i32[] [], x=w279) -> (*(type *) &x=w277:i32[])
        n90 = Swap Bytes(anything=w277) -> (byte swapped=w278:i32[])
        n91 = Swap Words(1:w278) -> (0:w271:i32[])
        n92 = Bundle By Name(cluster=w272, "nDim"=w271) -> (w273:T8)
        n93 = call <vilib>:"Add State(s) to Queue__jki_lib_state_machine.vi"("State(s) in (\"\")"=w282) -> ("States Out"=w281:string)  [unwired: 14 in]
      }
      frame "Parse: wData" {
        # "Convert from big endian to little endian for SGL"
        # "From the Igor Technical Document:\nwaveDataSize = wfmSize - offsetof(WaveHeader5, wData)\noffset of wData inside of WaveHeader5. This would be 320 (384-64)"
        # "Parse: wData\n(*)"
        n94 = Unbundle By Name(w293) -> ("Binary"=w299:string, "wfmSize"=w301:i32)
        n95 = Subtract(x=w301, y=320) -> (x-y=w297:i32)
        n96 = String Subset(string=w299, offset (0)=384, length (rest)=w297) -> (substring=w296:string)
        n97 = Type Cast(type=sgl[] [], x=w296) -> (*(type *) &x=w292:sgl[])
        n98 = Flatten To String(anything=w292, prepend array or string size? (T)=FALSE, byte order (0:big-endian, network order)=T7."big-endian, network order", error in (no error)=w285) -> (data string=w290:string, error out=w286:errorcluster)  [unwired: 1 out]
        n99 = Unflatten From String(type=w292, binary string=w290, data includes array or string size? (T)=FALSE, byte order (0:big-endian, network order)=T7."little-endian", error in (no error)=w286) -> (value=w291:sgl[], error out=w284:errorcluster)  [unwired: 1 out]
        n100 = Bundle By Name(cluster=w293, "wData"=w291) -> (w294:T8)
        n101 = call <vilib>:"Add State(s) to Queue__jki_lib_state_machine.vi"("State(s) in (\"\")"=w303) -> ("States Out"=w302:string)  [unwired: 14 in]
      }
      frame "Parse: Shape wData" {
        # "There are a lot of points\nDont want to duplicate data"
        # "Create array of zeros with dimensions i, j, k\nfor i in nDim[0]:\n     for j in nDim[1]:\n          for k in nDim[2]:\n               replace {zeros[i,j,k]} with wData[i+j+k]"
        # "256"
        # "256"
        # "4"
        # "256, 256, 4, 0"
        # "Parse: Shape wData\n(*)"
        n102 = Unbundle By Name(w310) -> ("nDim"=w315:i32[], "wData"=w308:sgl[])
        n103 = Index Array(array=w315) -> (element #1=w305:i32, element #2=w306:i32, element #3=w307:i32)  [unwired: 3 in]
        n104 = Initialize Array(sgl 0.0, w305, w306, w307) -> (w313:sgl[][][])
        n105 = for {
          N: w307 -> [_]
          tunnel: w306 -> [w326]
          tunnel: w305 -> [w325]
          shift-right: [w323] -> w304
          shift-left: w313 -> [w324]
          tunnel: w308 -> [w321]
          shift-right: [w319] -> _
          shift-left: 0 -> [w320]
          i -> [w322]
          n106 = for {
            N: w326 -> [_]
            tunnel: w325 -> [w334]
            shift-right: [w332] -> w323
            shift-left: w324 -> [w333]
            tunnel: w322 -> [w330]
            tunnel: w321 -> [w329]
            shift-right: [w327] -> w319
            shift-left: w320 -> [w328]
            i -> [w331]
            n107 = for {
              N: w334 -> [_]
              shift-right: [w342] -> w332
              shift-left: w333 -> [w343]
              tunnel: w331 -> [w340]
              tunnel: w330 -> [w339]
              tunnel: w329 -> [w338]
              shift-right: [w336] -> w327
              shift-left: w328 -> [w337]
              i -> [w341]
              n108 = Index Array(array=w338, index=w337) -> (element=w335:sgl)
              n109 = Replace Array Subset(array=w343, new element=w335, index (dim 0)=w341, index (dim 1)=w340, index (dim 2)=w339) -> (w342:sgl[][][])
              n110 = Increment(x=w337) -> (x+1=w336:i32)
            }
          }
        }
        n111 = Bundle By Name(cluster=w310, "wData"=sgl[] [], "Shaped wData"=w304) -> (w311:T8)
        n112 = call <vilib>:"Add State(s) to Queue__jki_lib_state_machine.vi"("State(s) in (\"\")"=w318) -> ("States Out"=w317:string)  [unwired: 14 in]
      }
      frame "Parse: Notes" {
        # "BinaryHeader5 size + wfmSize is the offset for the notes portion of the file."
        # "Parse: Notes\n(*)"
        n113 = Unbundle By Name(w345) -> ("Binary"=w351:string, "wfmSize"=w350:i32, "noteSize"=w347:i32)
        n114 = Add(x=w350, y=64) -> (x+y=w348:i32)
        n115 = String Subset(string=w351, offset (0)=w348, length (rest)=w347) -> (substring=w344:string)
        n116 = Bundle By Name(cluster=w345, "Notes"=w344) -> (w346:T8)
        n117 = call <vilib>:"Add State(s) to Queue__jki_lib_state_machine.vi"("State(s) in (\"\")"=w354) -> ("States Out"=w353:string)  [unwired: 14 in]
      }
      frame "---------- IMAQ ----------" {
        # "Template Separator\n(You can make a copy of, or modify, this frame)"
        n118 = call <vilib>:"Add State(s) to Queue__jki_lib_state_machine.vi"("State(s) in (\"\")"=w358) -> ("States Out"=w357:string)  [unwired: 14 in]
      }
      frame "IMAQ: Create" {
        # "Template Separator\n(You can make a copy of, or modify, this frame)"
        n119 = Unbundle By Name(w360) -> ("nDim"=w365:i32[], "Shaped wData"=w367:sgl[][][])
        n120 = Index Array(array=w365) -> (element #3=w366:i32)  [unwired: 3 in, 2 out]
        n121 = for {
          N: w366 -> [_]
          tunnel: [w376] -> w359 mode=indexing
          tunnel: w367 -> [w381]
          shift-right: [w377] -> w363
          shift-left: w364 -> [w378]
          tunnel: w362 -> [w379]
          i -> [w380]
          # "Flip to make it look right"
          # "Load array into IMAQ"
          # "Unique name for IMAQ Ref"
          n122 = Index Array(array=w381, index (dim 2)=w380) -> (element=w373:sgl[][])  [unwired: 2 in]
          n123 = Number To Decimal String(number=w380) -> (decimal integer string=w382:string)  [unwired: 1 in]
          n124 = Transpose 2D Array(2D array=w373) -> (transposed array=w374:sgl[][])
          n125 = call-poly <userlib>:"Reverse 2D Array__ogtk.vi"("by rows or columns (rows)"=enum16{"rows", "columns"}."rows", "Array"=w374) -> ("Reversed Array"=w372:sgl[][])  [unwired: 1 in]
          n126 = Concatenate Strings(w379, w382) -> ()  [unwired: 1 out]
          n127 = call "Convert Single to U8.vi"("Image Pixels (Float)"=w372) -> ("Image Pixels (U8)"=w370:u8[][])
          n128 = for {
            tunnel: w370 -> [w384] mode=indexing
            tunnel: [w383] -> w371 mode=indexing
            n129 = for {
              tunnel: w384 -> [w386] mode=indexing
              tunnel: [w385] -> w383 mode=indexing
              n130 = call <vilib>:"RGB to Color.vi"("B"=w386, "G"=w386, "R"=w386) -> ("Color"=w385:u32)
            }
          }
          n131 = New Data Value Reference(data value=w371, error in=w378) -> (data value reference=w376:refnum<data-value>, error out=w377:errorcluster)
        }
        n132 = Bundle By Name(cluster=w360, "Images"=w359) -> (w361:T8)
        n133 = call <vilib>:"Add State(s) to Queue__jki_lib_state_machine.vi"("State(s) in (\"\")"=w369) -> ("States Out"=w368:string)  [unwired: 14 in]
      }
      frame "---------- Notes ----------" {
        # "Template Separator\n(You can make a copy of, or modify, this frame)"
        n134 = call <vilib>:"Add State(s) to Queue__jki_lib_state_machine.vi"("State(s) in (\"\")"=w390) -> ("States Out"=w389:string)  [unwired: 14 in]
      }
      frame "Notes: Create LUT" {
        # "Notes: Create LUT\n(You can make a copy of, or modify, this frame)"
        n135 = Unbundle By Name(w398) -> ("Notes"=w397:string)
        n136 = call <vilib>:"Delimited String to 1D String Array.vi"("delimiter"="\r" ("Carriage Return Constant"), "delimited string"=w397) -> ("string array"=w396:string[])  [unwired: 9 in]
        n137 = for {
          tunnel: w396 -> [w411] mode=indexing
          shift-right: [w407] -> w393
          shift-left: variant -> [w406]
          shift-right: [w403] -> w392
          shift-left: w391 -> [w404]
          w408 = T10 1 items=["both", "start of string", "end of string"] ("location (both)")
          # "If the line is empty, dont write it to LUT"
          n138 = Match Pattern(string=w411, regular expression="\\:") -> (before substring=w402:string, after substring=w409:string)  [unwired: 1 in, 2 out]
          n139 = call <vilib>:"Trim Whitespace.vi"("string"=w409, "location (both)"=w408) -> ("trimmed string"=w401:string)
          n140 = Empty String/Path?(string/path=w402) -> (empty?=w405:bool)
          n141 = case shown="False" w405 {
            tunnel: [w417 w419] -> w407
            tunnel: w406 -> [w416 w419]
            tunnel: w401 -> [w415 _]
            tunnel: w402 -> [w414 _]
            tunnel: w404 -> [w413 w418]
            tunnel: [w412 w418] -> w403
            frame False {
              n142 = Set Variant Attribute(Variant=w416, name=w414, value=w415, error in=w413) -> (Variant out=w417:variant, error out=w412:errorcluster)  [unwired: 1 out]
            }
            frame True {
            }
          }
        }
        "Notes LUT" <- w393
        n143 = call <vilib>:"Add State(s) to Queue__jki_lib_state_machine.vi"("State(s) in (\"\")"=w400) -> ("States Out"=w399:string)  [unwired: 14 in]
      }
      frame "---------- Directory ----------" {
        # "Template Separator\n(You can make a copy of, or modify, this frame)"
        n144 = call <vilib>:"Add State(s) to Queue__jki_lib_state_machine.vi"("State(s) in (\"\")"=w423) -> ("States Out"=w422:string)  [unwired: 14 in]
      }
      frame "Directory: Bin Header" {
        # "This is a key for the string lengths and Indices of all of the values in the bin header"
        # "Length|Index|typedef struct BinHeader5 {\n     2|    0|\tshort version;\t\t\t\t\t\t          // Version number for backwards compatibility.\n     2|    2|\tshort checksum;\t\t\t\t\t\t         // Checksum over this header and the wave header.\n     4|    4|\tlong wfmSize;\t\t\t\t\t\t           // The size of the WaveHeader5 data structure plus the wave data.\n     4|    8|\tlong formulaSize;\t\t\t\t\t        // The size of the dependency formula, if any.\n     4|   12|\tlong noteSize;\t\t\t\t\t\t          // The size of the note text.\n     4|   16|\tlong dataEUnitsSize;\t\t\t\t      // The size of optional extended data units.\n    16|   20|\tlong dimEUnitsSize[MAXDIMS];\t\t// The size of optional extended dimension units.\n    16|   36|\tlong dimLabelsSize[MAXDIMS];\t\t// The size of optional dimension labels.\n     4|   52|\tlong sIndicesSize;\t\t\t\t\t       // The size of string indicies if this is a text wave.\n     4|   56|\tlong optionsSize1;\t\t\t\t\t       // Reserved. Write zero. Ignore on read.\n     4|   60|\tlong optionsSize2;\t\t\t\t\t       // Reserved. Write zero. Ignore on read.\n      |   64|} BinHeader5;"
        n145 = call <vilib>:"Add State(s) to Queue__jki_lib_state_machine.vi"("State(s) in (\"\")"=w427) -> ("States Out"=w426:string)  [unwired: 14 in]
      }
      frame "Directory: Wave Header" {
        # "Expand to see all documentation"
        # "Length|Index|struct WaveHeader5 {\n     4|   64|\tstruct WaveHeader5 **next;\t\t\t  // link to next wave in linked list.\n     4|   68|\tunsigned long creationDate;\t\t \t// DateTime of creation.\n     4|   72|\tunsigned long modDate;\t\t\t\t     // DateTime of last modification.\n     4|   76|\tlong npnts;\t\t\t\t\t\t\t             // Total number of points (multiply dimensions up to first zero).\n     2|   80|\tshort type;\t\t\t\t\t\t\t             // See types (e.g. NT_FP64) above. Zero for text waves.\n     2|   82|\tshort dLock;\t\t\t\t\t\t             // Reserved. Write zero. Ignore on read.\n     6|   84|\tchar whpad1[6];\t\t\t\t\t\t          // Reserved. Write zero. Ignore on read.\n     2|   90|\tshort whVersion;\t\t\t\t\t          // Write 1. Ignore on read.\n    32|   92|\tchar bname[MAX_WAVE_NAME5+1];\t\t// Name of wave plus trailing null.\n     4|  124|\tlong whpad2;\t\t\t\t\t\t             // Reserved. Write zero. Ignore on read.\n     4|  128|\tstruct DataFolder **dFolder;\t\t // Used in memory only. Write zero. Ignore on read.\n      |     |\t// Dimensioning info. [0] == rows, [1] == cols etc\n    16|  132|\tlong nDim[MAXDIMS];\t\t\t\t\t       // Number of of items in a dimension -- 0 means no data.\n    32|  148|\tdouble sfA[MAXDIMS];\t\t\t\t       // Index value for element e of dimension d = sfA[d]*e + sfB[d].\n    32|  180|\tdouble sfB[MAXDIMS];\n      |     |\t// SI units\n     4|  212|\tchar dataUnits[MAX_UNIT_CHARS+1];\t\t\t      // Natural data units go here - null if none.\n    16|  216|\tchar dimUnits[MAXDIMS][MAX_UNIT_CHARS+1];\t// Natural dimension units go here - null if none.\n     2|  232|\tshort fsValid;\t\t\t\t\t\t                      // TRUE if full scale values have meaning.\n     2|  234|\tshort whpad3;\t\t\t\t\t\t                       // Reserved. Write zero. Ignore on read.\n    16|  236|\tdouble topFullScale,botFullScale;\t        // The max and max full scale value for wave.\n     4|  252|\tHandle dataEUnits;\t\t\t\t\t                   // Used in memory only. Write zero. Ignore on read.\n    16|  256|\tHandle dimEUnits[MAXDIMS];\t\t\t             // Used in memory only. Write zero. Ignore on read.\n    16|  272|\tHandle dimLabels[MAXDIMS];\t\t\t             // Used in memory only. Write zero. Ignore on read.\n     4|  288|\tHandle waveNoteH;\t\t\t\t\t                    // Used in memory only. Write zero. Ignore on read.\n    64|  292|\tlong whUnused[16];\t\t\t\t\t                   // Reserved. Write zero. Ignore on read.\n      |     |\t// The following stuff is considered private to Igor.\n     2|  356|\tshort aModified;\t\t\t\t\t                     // Used in memory only. Write zero. Ignore on read.\n     2|  358|\tshort wModified;\t\t\t\t\t                     // Used in memory only. Write zero. Ignore on read.\n     2|  360|\tshort swModified;\t\t\t\t\t                    // Used in memory only. Write zero. Ignore on read.\n     1|  362|\tchar useBits;\t\t\t\t\t\t                       // Used in memory only. Write zero. Ignore on read.\n     1|  363|\tchar kindBits;\t\t\t\t\t\t                      // Reserved. Write zero. Ignore on read.\n     4|  364|\tvoid **formula;\t\t\t\t\t\t                     // Used in memory only. Write zero. Ignore on read.\n     4|  368|\tlong depID;\t\t\t\t\t\t\t                        // Used in memory only. Write zero. Ignore on read.\n     2|  372|\tshort whpad4;\t\t\t\t\t\t                       // Reserved. Write zero. Ignore on read.\n     2|  374|\tshort srcFldr;\t\t\t\t\t\t                      // Used in memory only. Write zero. Ignore on read.\n     4|  376|\tHandle fileName;\t\t\t\t\t                     // Used in memory only. Write zero. Ignore on read.\n     4|  380|\tlong **sIndices;\t\t\t\t\t                     // Used in memory only. Write zero. Ignore on read.\n     4|  384|\tfloat wData[1];\t\t\t\t\t\t                     // The start of the array of data. Must be 64 bit aligned.\n      |  388|};"
        # "This is a key for the string lengths and Indices of all of the values in the wave header"
        n146 = call <vilib>:"Add State(s) to Queue__jki_lib_state_machine.vi"("State(s) in (\"\")"=w431) -> ("States Out"=w430:string)  [unwired: 14 in]
      }
    }
  }
  "error out" <- w20
  n147 = Unbundle By Name(w17) -> ("Images"=w16:refnum<data-value>[])
  n148 = for {
    tunnel: w16 -> [w436] mode=indexing
    tunnel: [w435] -> w15 mode=indexing
    tunnel: [w432] -> w11 mode=indexing
    n149 = in-place {
      n150 = in-place-dvr #1(w436) -> (w437:u32[][])  [unwired: 1 out]
      n151 = in-place-dvr #1(w437) -> (w432:refnum<data-value>)  [unwired: 1 out]
    }
    n152 = call <vilib>:"Draw Multiple Lines.vi"("line endpoints"=cluster{"x":i16, "y":i16}[] [{"x"=0, "y"=100}, {"x"=100, "y"=0}], "color(black)"=u32 14417948) -> ("new picture"=w435:picture)  [unwired: 7 in]
  }
  "Array" <- w15
  n153 = New Data Value Reference(data value=u32[][] []) -> (data value reference=w13:refnum<data-value>)  [unwired: 1 in, 1 out]
  n154 = Index Array(array=w11) -> (element=w14:refnum<data-value>)  [unwired: 1 in]
  n155 = in-place {
    n156 = in-place-dvr #2(w14) -> (w438:u32[][])  [unwired: 1 out]
    n157 = in-place-dvr #3(w13) -> ()  [unwired: 2 out]
    n158 = in-place-dvr #2(w438) -> (w9:errorcluster)  [unwired: 1 out]
    n159 = in-place-dvr #3(w438) -> (w12:refnum<data-value>)  [unwired: 1 out]
  }
  n160 = control-ref of="new picture"() -> (w7:refnum<vi>)
  n161 = property class="Pict"(reference=w7, "ZoomFactor"=sgl 0.5 ("Zoom Factor"), "Draw Area Size"=T2 {"Width"=256, "Height"=256}, "Origin"=T3 {"Horizontal"=0, "Vertical"=0}) -> (error out=w3:errorcluster)  [unwired: 1 in, 1 out]
  n162 = in-place {
    in-place-border: w3 -> [_]
    in-place-border: [w447] -> w1
    n163 = in-place-dvr #4(w12) -> (w456:u32[][])  [unwired: 1 out]
    n164 = call-poly <vilib>:"Draw Unflattened Pixmap.vi"("data (RGB format)"=w456) -> ("new picture"=w454:picture)  [unwired: 8 in]
    n165 = call <vilib>:"Picture to Pixmap.vi"("picture"=w454) -> ("image data"=w449:T11)  [unwired: 9 in, 1 out]
    n166 = Unbundle By Name(w449) -> ("image"=w448:u8[])
    n167 = Array Size(array=w448) -> (size(s)=→"size(s) 3":i32)
    n168 = call-poly <vilib>:"Resize Image.vi"("Scale"=10.0, "Image"=w449) -> ("Resized Image"=w453:T11)  [unwired: 8 in, 1 out]
    n169 = Unbundle By Name(w453) -> ("image"=w452:u8[])
    n170 = call <vilib>:"Draw Flattened Pixmap.vi"("image data"=w453) -> ("new picture"=w446:picture)  [unwired: 8 in]
    n171 = Array Size(array=w452) -> (size(s)=→"size(s) 2":i32)
    n172 = call <vilib>:"Draw Circle by Radius.vi"("color(black)"=u32 14417948, "pixel center"=cluster{"horizontal":i16, "vertical":i16} {"horizontal"=300, "vertical"=300}, "radius"=i16 300, "picture"=w446) -> ("new picture"=w441:picture)  [unwired: 7 in]
    n173 = call "Empty Picture"() -> ()  [unwired: 1 out]
    n174 = call <vilib>:"Draw Multiple Lines.vi"("picture"=w441, "line endpoints"=cluster{"x":i16, "y":i16}[] [{"x"=10, "y"=0}, {"x"=20, "y"=20}, {"x"=50, "y"=75}, {"x"=100, "y"=10}, {"x"=0, "y"=200}], "color(black)"=u32 16711681) -> ("new picture"=w440:picture)  [unwired: 6 in]
    n175 = Concatenate Strings(w440) -> (w447:picture)
    "new picture" <- w447
    n176 = in-place-dvr #4(w456) -> (w10:refnum<data-value>)  [unwired: 1 out]
  }
  n177 = for {
    tunnel: w11 -> [w457] mode=indexing
    tunnel: w9 -> [_]
    n178 = Delete Data Value Reference(data value reference=w457) -> ()  [unwired: 1 in, 2 out]
  }
  n179 = Delete Data Value Reference(data value reference=w10) -> (error out=w2:errorcluster)  [unwired: 1 in, 1 out]
  n180 = disable-structure shown="Enabled" {
    disable-tunnel: w2 -> [w459 _]
    disable-tunnel: w1 -> [w458 _]
    frame Enabled {
      # "Image is loaded from file into arrays\nDVRs are created\nCopy"
      n181 = call <vilib>:"Add State(s) to Queue__jki_lib_state_machine.vi"("State(s) in (\"\")"="Macro: Initialize") -> ("States Out"=w462:string)  [unwired: 14 in]
      n182 = while "JKI State Machine 2018" {
        shift-right: [w467] -> _
        shift-left: _ -> [w466]
        shift-right: [w470] -> _
        shift-left: w459 -> [w464]
        shift-right: [w469] -> _
        shift-left: w462 -> [w471]
        tunnel: "Selection" -> [w463]
        stop <- w468 stop-if-true
        w465 = -1  # Timeout
        # "Template Copyright © 2018 JKI - http://jki.net/state-machine"
        n183 = call <vilib>:"Parse State Queue__jki_lib_state_machine.vi"("State Queue"=w471, "Error In (no error)"=w464) -> ("Remaining States"=w473:string, "Current State"=w474:string, "Arguments"=w472:string)  [unwired: 11 in]
        n184 = case shown="\"\", \"Event Structure\", \"Idle\"" w474 {
          selector: w474 -> [_ _ w562 _ _ _ _ _ _ _ _ _ _ _ _ _ _ _ _]
          tunnel: w473 -> [w481 w561 w566 w585 w591 w596 w600 w610 w616 w620 w627 w633 w644 w713 w718 w728 w732 w744 w748]
          tunnel: w472 -> [_ _ _ _ _ _ _ _ _ _ _ w628 w638 _ _ _ _ _ _]
          tunnel: w466 -> [w479 w558 w564 w578 w588 w594 w597 _ w611 w617 w625 w631 w640 w710 w715 w725 w729 w741 w745]
          tunnel: [w478 w559 w568 w582 errorcluster {"status"=FALSE, "code"=0, "source"=""} ("error out") w593 w598 w607 w612 w618 w624 w629 w641 w711 w716 w726 w730 w742 w746] -> w470
          tunnel: w464 -> [w477 w559 w567 w582 w587 w593 w598 w607 w613 w618 w624 w630 w642 w711 w716 w726 w730 w742 w746]
          tunnel: [w480 w560 w565 w584 w590 w595 w599 w609 w615 w619 w626 w632 w643 w712 w717 w727 w731 w743 w747] -> w469
          tunnel: [_ _ _ _ _ TRUE _ _ _ _ _ _ _ _ _ _ _ _ _] -> w468
          tunnel: [w476 w558 w564 w583 w588 w594 w597 w608 w611 w617 w625 w631 w640 w710 w715 w725 w729 w741 w745] -> w467
          tunnel: w465 -> [w475 _ _ _ _ _ _ _ _ _ _ _ _ _ _ _ _ _ _]
          tunnel: w463 -> [_ _ _ _ _ _ _ w601 _ _ _ _ _ _ _ _ _ _ _]
          frame "", "Event Structure", "Idle" {
            # "executes when the state queue is empty"
            n185 = event shown="[6] Panel Close?" {
              selector: _ -> [_ _ _ _ _ _ _]
              dyn-events: _ -> [_ _ _ _ _ _ _]
              timeout: w475 -> [_ _ _ _ _ _ _]
              tunnel: w481 -> [w485 w491 w505 w522 w528 w542 w557]
              tunnel: [w484 w490 w504 w521 w527 w541 w556] -> w480
              tunnel: w479 -> [w482 w487 w502 w517 w524 w537 w554]
              tunnel: [w483 w489 w503 w520 w526 w540 w555] -> w478
              tunnel: w477 -> [w483 w489 w503 w520 w526 w540 w555]
              tunnel: [w482 w488 w500 w518 w525 w539 w554] -> w476
              event Timeout {
                # "Timeout Frame\n(this will only execute if the Event Structure timeout is >= 0)"
                n186 = event-data() -> ()  [unwired: 1 in, 1 out]
                n187 = call <vilib>:"Add State(s) to Queue__jki_lib_state_machine.vi"("State(s) in (\"\")"=w485) -> ("States Out"=w484:string)  [unwired: 14 in]
              }
              event "Selection": Value Change {
                # "Timeout Frame\n(this will only execute if the Event Structure timeout is >= 0)"
                n188 = event-data() -> ("NewVal"=w486:T1)  [unwired: 1 in, 5 out]
                "NewVal" <- w486
                n189 = Bundle By Name(cluster=w487, "Selection"=w486) -> (w488:T12)
                n190 = call <vilib>:"Add State(s) to Queue__jki_lib_state_machine.vi"("State(s) in (\"\")"=w491) -> ("States Out"=w490:string)  [unwired: 14 in]
              }
              event "2D Picture": Mouse Down {
                (unwired) TRUE ("MD")
                # "Timeout Frame\n(this will only execute if the Event Structure timeout is >= 0)"
                n191 = event-data() -> ("CtlRef"=w495:refnum<vi>, "Coords"=w499:T4, "Button"=→"Button":u16, "Mods.Double Click"=w496:bool, "PlatMods.Ctrl"=w493:bool)  [unwired: 1 in, 3 out]
                n192 = property class="Pict"(reference=w495) -> ("Origin"=w498:T3, "ZoomFactor"=w492:sgl)  [unwired: 1 in, 2 out]
                n193 = case shown="True" w496 {
                  tunnel: w495 -> [_ w515]
                  tunnel: w492 -> [_ w511]
                  tunnel: w493 -> [_ w513]
                  frame False {
                  }
                  frame True {
                    n194 = Increment(x=w511) -> (x+1=w514:sgl)
                    n195 = Decrement(x=w511) -> (x-1=w512:sgl)
                    n196 = Select(t=w512, s=w513, f=w514) -> (s? t:f=w507:sgl)
                    n197 = Less Or Equal To 0?(x=w507) -> (x <= 0?=w508:bool)
                    n198 = Divide(x=w511, y=sgl 2.0) -> (x/y=w509:sgl)
                    n199 = Select(t=w509, s=w508, f=w507) -> (s? t:f=w506:sgl)
                    n200 = property class="Pict"(reference=w515, "ZoomFactor"=w506) -> ()  [unwired: 1 in, 2 out]
                  }
                }
                n201 = Not(x=w496) -> (.not. x?=w497:bool)
                n202 = Bundle By Name(cluster=w502, "MD Coords"=w499, "MD"=w497) -> (w501:T12)
                n203 = Bundle By Name(cluster=w501, "MD Origin"=w498) -> (w500:T12)
                n204 = call <vilib>:"Add State(s) to Queue__jki_lib_state_machine.vi"("State(s) in (\"\")"=w505) -> ("States Out"=w504:string)  [unwired: 14 in]
              }
              event "2D Picture": Mouse Up {
                # "Timeout Frame\n(this will only execute if the Event Structure timeout is >= 0)"
                n205 = event-data() -> ("Coords"=w519:T4)  [unwired: 1 in, 7 out]
                n206 = Bundle By Name(cluster=w517, "MU Coords"=w519, "MD"=FALSE) -> (w518:T12)
                n207 = call <vilib>:"Add State(s) to Queue__jki_lib_state_machine.vi"("State(s) in (\"\")"=w522) -> ("States Out"=w521:string)  [unwired: 14 in]
              }
              event "2D Picture": Mouse Leave {
                # "Timeout Frame\n(this will only execute if the Event Structure timeout is >= 0)"
                n208 = event-data() -> ()  [unwired: 1 in, 4 out]
                n209 = Bundle By Name(cluster=w524, "MD"=FALSE) -> (w525:T12)
                n210 = call <vilib>:"Add State(s) to Queue__jki_lib_state_machine.vi"("State(s) in (\"\")"=w528) -> ("States Out"=w527:string)  [unwired: 14 in]
              }
              event "2D Picture": Mouse Move {
                # "Timeout Frame\n(this will only execute if the Event Structure timeout is >= 0)"
                n211 = event-data() -> ("CtlRef"=w532:refnum<vi>, "Coords"=w535:T4)  [unwired: 1 in, 3 out]
                n212 = Unbundle By Name(w537) -> ("MD Coords"=w536:T4, "MD Origin"=w534:T4, "MD"=w538:bool)
                n213 = Subtract(x=w536, y=w535) -> (x-y=w530:T4)
                n214 = property class="Pict"(reference=w532) -> ("ZoomFactor"=w531:sgl)  [unwired: 1 in, 2 out]
                n215 = Divide(x=w530, y=w531) -> (x/y=w529:cluster{"Horizontal":sgl, "Vertical":sgl})
                n216 = Add(x=w529, y=w534) -> (x+y=w533:cluster{"Horizontal":sgl, "Vertical":sgl})
                n217 = case shown="True" w538 {
                  tunnel: w533 -> [_ w546]
                  tunnel: w532 -> [_ w550]
                  frame False {
                  }
                  frame True {
                    n218 = property class="Pict"(reference=w550) -> (reference out=w551:refnum<vi>, "Origin"=→"Origin":T3, "Draw Area Size"=w544:T2)  [unwired: 1 in, 1 out]
                    "Draw Area Size" <- w544
                    n219 = Subtract(x=cluster{"Horizontal":sgl, "Vertical":sgl} {"Horizontal"=1024.0, "Vertical"=1024.0} ("upper limit"), y=w544) -> (x-y=w543:cluster{sgl, sgl})
                    n220 = In Range and Coerce(upper limit=w543, x=w546, lower limit=cluster{"Horizontal":sgl, "Vertical":sgl} {"Horizontal"=0.0, "Vertical"=0.0}) -> (coerced(x)=w547:cluster{"Horizontal":sgl, "Vertical":sgl})  [unwired: 1 out]
                    n221 = property class="Pict"(reference=w551, "Origin"=w547) -> ()  [unwired: 1 in, 2 out]
                  }
                }
                n222 = Bundle By Name(cluster=w537, "MU Coords"=w535) -> (w539:T12)
                n223 = call <vilib>:"Add State(s) to Queue__jki_lib_state_machine.vi"("State(s) in (\"\")"=w542) -> ("States Out"=w541:string)  [unwired: 14 in]
              }
              event Panel Close? {
                # "Discard the event because we'll close the front panel ourselves in Macro: Exit"
                # "Close Panel button (pressed) Event\n(this executes Macro: Exit to terminate the VI)"
                n224 = event-data() -> ()  [unwired: 1 in, 1 out]
                n225 = event-data("Discard?"=TRUE) -> ()  [unwired: 1 in, 1 out]
                n226 = call <vilib>:"Add State(s) to Queue__jki_lib_state_machine.vi"("State(s) in Front (\"\")"="Macro: Exit", "State(s) in (\"\")"=w557) -> ("States Out"=w556:string)  [unwired: 13 in]
              }
            }
          }
          frame "---------- Core ----------" {
            # "Do not put any code in this frame.\n(it is a separator no-op)"
            n227 = call <vilib>:"Add State(s) to Queue__jki_lib_state_machine.vi"("State(s) in (\"\")"=w561) -> ("States Out"=w560:string)  [unwired: 14 in]
          }
          frame Default {
            w571 = 42 items=["No error", "Argument error", "Memory is full", "Out of zone", "End of file", "File already open", "Generic file I/O error", "File not found", "File permission error", "Disk is full", "Duplicate path", "Too many files open", "System feature not enabled", "Resource file not found", "Cannot add resource", "Resource not found", "Image not found", "Image memory error", "Pen does not exist", "Config type invalid", "Config token not found", "Config parse error", "Config memory error", "Bad external code format", "Bad external code offset", "External code not present", "Null window", "Destroy window error", "Null menu", "Print aborted", "Bad print record", "Print driver error", "Windows error during printing", "Memory error during printing", "Print dialog error", "Generic print error", "Invalid device refnum", "Device not found", "Device parameter error", "Device unit error", "Cannot open device", "Device call aborted", "Generic error", "Cancelled by user", "Object ID too low", "Object ID too high", "Object not in heap", "Unknown heap", "Unknown object (invalid DefProc)", "Unknown object (DefProc not in table)", "Message out of range", "Invalid (null) method", "Unknown message", "Manager call not supported", "Bad address", "Network operation in progress", "Network operation timed out", "Connection is busy", "Network attribute not supported", "Network error", "Address in use", "System out of memory", "Connection aborted", "Connection refused", "Not connected", "Already connected", "Connection closed", "Initialization error (interapplication manager)", "Bad occurrence", "Wait on unbound occurrence handler", "Occurrence queue overflow", "Datalog type conflict", "Unused", "Unrecognized type (interapplication manager)", "Memory corrupt", "Failed to make temporary DLL", "Old CIN version", "Drag socket not found", "Failed to load drop-object", "Failed to register OLE object", "Failed to release OLE object", "Format specifier type mismatch", "Unknown format specifier", "Too few format specifiers", "Too many format specifiers", "Scan failed", "Newer CIN version", "Error converting to variant", "Runtime menu error", "Password tampered", "Variant attribute not found", "Incompatible variant data type", "Event data is not available", "Event Store is not present", "Occurrence is not found", "Event Queue is not created", "Event info is not available", "Refnum passed is NULL", "Error retrieving Class GUID", "Error retrieving CoClass GUID", "Error retrieving TypeLib GUID.", "Bad built application magic bytes.", "Specific driver is different from the specific driver associated with the Logical Name.", "There is no session opened to the class driver.", "Max Error", "MAX - Error with config objects", "MAX - Error loading configuration", "MAX - Group not supported"]
            # "State Syntax:\nStateCategory: State >> Argument\nLine Terminator: Line feed\nExample:\nUI: Help >> About\n\nWhere \"UI\" is the state category\nWhere \"Help\" is the state\nWhere \"About\" is the argument\nOther Examples:\nApp Data: Initialize\nUI: Initialize\nHelp >> About\n\nCommenting:\nTo add a comment use \"//\" or \"#\" and all text to the right will be ignored\nCommenting Example:\nUI: Initialize // This initializes the UI\n# This whole line is a comment\n// Another comment line"
            # "Current State"
            # "Do not delete, rename, or modify this frame.\n(this is used to capture unhandled states and typos)"
            # "Handle mistyped state name (developer tool)"
            n228 = Format Into String(format string="Software Exception: Unhandled State \"%s\"." ("message"), error in=w567, w562) -> (resulting string=w570:string, error out=w569:errorcluster)  [unwired: 1 in]
            n229 = call <vilib>:"Error Cluster From Error Code.vi"("show call chain? (False)"=TRUE, "error in (no error)"=w569, "error message (\"\")"=w570, "error code (0)"=w571) -> ("error out"=w568:errorcluster)  [unwired: 5 in]
            n230 = call <vilib>:"Add State(s) to Queue__jki_lib_state_machine.vi"("State(s) in (\"\")"=w566) -> ("States Out"=w565:string)  [unwired: 14 in]
          }
          frame "Initialize Core Data" {
            # "Do not delete, rename, or modify this frame.\n(this is used to determine panel behavior on exit)"
            # "originally closed?"
            # "exe?"
            # "If panel starts closed or is an EXE, then close it when we exit"
            n231 = property class="VI"() -> ("FP.State"=w575:T5)  [unwired: 2 in, 2 out]
            n232 = property class="App"() -> ("App.Kind"=w581:T6)  [unwired: 2 in, 2 out]
            n233 = control-ref of="Current VI Reference"() -> (w576:refnum<vi>)
            n234 = Equal?(x=w575, y=T5."Closed" ("Front Panel Window:State")) -> (x = y?=w573:bool)
            n235 = Equal?(x=w581, y=T6."Run Time System" ("Application:Kind")) -> (x = y?=w579:bool)
            n236 = Or(x=w573, y=w579) -> (x .or. y?=w577:bool)
            n237 = Bundle By Name(cluster=w578, "Core.Current VI Reference"=w576, "Core.Close Panel on Exit?"=w577) -> (w583:T12)
            n238 = call <vilib>:"Add State(s) to Queue__jki_lib_state_machine.vi"("State(s) in (\"\")"=w585) -> ("States Out"=w584:string)  [unwired: 14 in]
          }
          frame "Error Handler" {
            # "Unhandled Error -- Display it"
            # "Handle any errors here.\nYou can also output any states to clean-up after errors occur"
            # "Clear error"
            n239 = call <vilib>:"General Error Handler.vi"("error in (no error)"=w587) -> ()  [unwired: 10 in, 5 out]
            n240 = call <vilib>:"Add State(s) to Queue__jki_lib_state_machine.vi"("State(s) in Front (\"\")"="/* Post Error States", "State(s) in (\"\")"=w591) -> ("States Out"=w590:string)  [unwired: 13 in]
          }
          frame "Exit" {
            # "Do not put any code in this frame.\n(No errors that occur here will be handled.)"
            n241 = call <vilib>:"Add State(s) to Queue__jki_lib_state_machine.vi"("State(s) in (\"\")"=w596) -> ("States Out"=w595:string)  [unwired: 14 in]
          }
          frame "---------- Data ----------" {
            # "Do not put any code in this frame.\n(It is a separator no-op. You can make a copy of this frame to create a new Data frame)"
            n242 = call <vilib>:"Add State(s) to Queue__jki_lib_state_machine.vi"("State(s) in (\"\")"=w600) -> ("States Out"=w599:string)  [unwired: 14 in]
          }
          frame "Data: Initialize" {
            w602 = T4 {"Horizontal"=0, "Vertical"=0}  # MD Origin
            w603 = FALSE  # MD
            w604 = T4 {"Horizontal"=0, "Vertical"=0}  # MU Coords
            w605 = T4 {"Horizontal"=0, "Vertical"=0}  # MD Coords
            w606 = T9 {"Current VI Reference"=refnum, "Close Panel on Exit?"=FALSE}  # Core
            # "do not delete - used by framework"
            # "Data names and types of shift register data are defined by this bundle."
            # "Initialize the shift-register data, here.\n(data names are defined by what you wire into the bundle function)"
            n243 = Bundle("Core"=w606, "MD Coords"=w605, "MU Coords"=w604, "MD"=w603, "MD Origin"=w602, "Selection"=w601) -> (w608:T12)  [unwired: 1 in]
            n244 = call <vilib>:"Add State(s) to Queue__jki_lib_state_machine.vi"("State(s) in (\"\")"=w610) -> ("States Out"=w609:string)  [unwired: 14 in]
          }
          frame "Data: Cleanup" {
            # "Cleanup any data and references, here.\n(this is called automatically, by the Macro: Exit)"
            n245 = Unbundle By Name(w611) -> ("Core.Current VI Reference"=w614:refnum<vi>)
            n246 = Close Reference(reference=w614, error in (no error)=w613) -> (error out=w612:errorcluster)
            n247 = call <vilib>:"Add State(s) to Queue__jki_lib_state_machine.vi"("State(s) in (\"\")"=w616) -> ("States Out"=w615:string)  [unwired: 14 in]
          }
          frame "---------- UI ----------" {
            # "Do not put any code in this frame.\n(It is a separator no-op. You can make a copy of this frame to create a new UI frame)"
            n248 = call <vilib>:"Add State(s) to Queue__jki_lib_state_machine.vi"("State(s) in (\"\")"=w620) -> ("States Out"=w619:string)  [unwired: 14 in]
          }
          frame "UI: Initialize" {
            # "Initialize the User Interface, here.\n(this is called automatically, by the Macro: Init)"
            n249 = control-ref of="2D Picture"() -> (w623:refnum<vi>)
            n250 = property class="Pict"(reference=w623, "Origin"=T3 {"Horizontal"=0, "Vertical"=0}, "ZoomFactor"=sgl 1.0 ("Zoom Factor")) -> ()  [unwired: 1 in, 2 out]
            n251 = call <vilib>:"Add State(s) to Queue__jki_lib_state_machine.vi"("State(s) in (\"\")"=w627) -> ("States Out"=w626:string)  [unwired: 14 in]
          }
          frame "UI: Cursor Set" {
            # "Argument"
            # "Set and Unset Cursor Busy.\n(Usage: \"UI: Cursor Set >> Busy|Idle\")"
            n252 = case shown="\"Idle\", Default" w628 {
              tunnel: w630 -> [w635 w637]
              tunnel: [w634 w636] -> w629
              frame "Idle", Default {
                n253 = call <vilib>:"Unset Busy.vi"("error in (no error)"=w635) -> ("error out"=w634:errorcluster)  [unwired: 10 in]
              }
              frame "Busy" {
                n254 = call <vilib>:"Set Busy.vi"("error in (no error)"=w637) -> ("error out"=w636:errorcluster)  [unwired: 9 in, 1 out]
              }
            }
            n255 = call <vilib>:"Add State(s) to Queue__jki_lib_state_machine.vi"("State(s) in (\"\")"=w633) -> ("States Out"=w632:string)  [unwired: 14 in]
          }
          frame "UI: Front Panel State" {
            # "Argument"
            # "Set Front Panel Open or Closed\n(Usage: \"UI: Front Panel State >> Open|Close\")"
            n256 = Unbundle By Name(w640) -> ("Core.Current VI Reference"=w639:refnum<vi>)
            n257 = case shown="\"Minimize\", \"Minimized\"" w638 {
              tunnel: w642 -> [w650 w665 w676 w689 w702]
              tunnel: [w652 w666 w678 w691 w704] -> w641
              tunnel: w639 -> [w651 w663 w677 w690 w703]
              frame "Open", "Standard", Default {
                w645 = T5."Standard" ("State")
                n258 = property class="VI"(reference=w651, error in=w650) -> (reference out=w648:refnum<vi>, error out=w649:errorcluster, "FP.State"=w647:T5)
                n259 = Not Equal?(x=w647, y=w645) -> (x != y?=w646:bool)
                n260 = case shown="True" w646 {
                  tunnel: [w656 w658] -> w652
                  tunnel: w649 -> [w655 w658]
                  tunnel: w648 -> [w654 _]
                  tunnel: w645 -> [w653 _]
                  frame True {
                    n261 = invoke class="VI" method="FP.Open"(reference=w654, error in=w655, "Activate"=TRUE, "State"=w653) -> (error out=w656:errorcluster)  [unwired: 1 in, 4 out]
                  }
                  frame False {
                  }
                }
              }
              frame "Close", "Closed" {
                n262 = property class="VI"(reference=w663, error in=w665) -> (reference out=w662:refnum<vi>, error out=w664:errorcluster, "FP.State"=w660:T5)
                n263 = Not Equal?(x=w660, y=T5."Closed" ("Front Panel Window:State")) -> (x != y?=w659:bool)
                n264 = case shown="True" w659 {
                  tunnel: [w667 w670] -> w666
                  tunnel: w664 -> [w667 w669]
                  tunnel: w662 -> [_ w668]
                  frame False {
                  }
                  frame True {
                    n265 = invoke class="VI" method="FP.Close"(reference=w668, error in=w669) -> (error out=w670:errorcluster)  [unwired: 1 in, 2 out]
                  }
                }
              }
              frame "Hidden", "Hide" {
                w671 = T5."Hidden" ("State")
                n266 = property class="VI"(reference=w677, error in=w676) -> (reference out=w674:refnum<vi>, error out=w675:errorcluster, "FP.State"=w673:T5)
                n267 = Not Equal?(x=w673, y=w671) -> (x != y?=w672:bool)
                n268 = case shown="True" w672 {
                  tunnel: [w682 w683] -> w678
                  tunnel: w675 -> [w681 w683]
                  tunnel: w674 -> [w680 _]
                  tunnel: w671 -> [w679 _]
                  frame True {
                    n269 = invoke class="VI" method="FP.Open"(reference=w680, error in=w681, "State"=w679) -> (error out=w682:errorcluster)  [unwired: 2 in, 4 out]
                  }
                  frame False {
                  }
                }
              }
              frame "Minimize", "Minimized" {
                w684 = T5."Minimized" ("State")
                n270 = property class="VI"(reference=w690, error in=w689) -> (reference out=w687:refnum<vi>, error out=w688:errorcluster, "FP.State"=w686:T5)
                n271 = Not Equal?(x=w686, y=w684) -> (x != y?=w685:bool)
                n272 = case shown="True" w685 {
                  tunnel: [w695 w696] -> w691
                  tunnel: w688 -> [w694 w696]
                  tunnel: w687 -> [w693 _]
                  tunnel: w684 -> [w692 _]
                  frame True {
                    n273 = invoke class="VI" method="FP.Open"(reference=w693, error in=w694, "State"=w692) -> (error out=w695:errorcluster)  [unwired: 2 in, 4 out]
                  }
                  frame False {
                  }
                }
              }
              frame "Maximize", "Maximized" {
                w697 = T5."Maximized" ("State")
                n274 = property class="VI"(reference=w703, error in=w702) -> (reference out=w700:refnum<vi>, error out=w701:errorcluster, "FP.State"=w699:T5)
                n275 = Not Equal?(x=w699, y=w697) -> (x != y?=w698:bool)
                n276 = case shown="True" w698 {
                  tunnel: [w708 w709] -> w704
                  tunnel: w701 -> [w707 w709]
                  tunnel: w700 -> [w706 _]
                  tunnel: w697 -> [w705 _]
                  frame True {
                    n277 = invoke class="VI" method="FP.Open"(reference=w706, error in=w707, "State"=w705) -> (error out=w708:errorcluster)  [unwired: 2 in, 4 out]
                  }
                  frame False {
                  }
                }
              }
            }
            n278 = call <vilib>:"Add State(s) to Queue__jki_lib_state_machine.vi"("State(s) in (\"\")"=w644) -> ("States Out"=w643:string)  [unwired: 14 in]
          }
          frame "---------- Macro ----------" {
            # "Do not put any code in this frame.\n(It is a separator no-op. You can make a copy of this frame to create a new Macro frame)"
            n279 = call <vilib>:"Add State(s) to Queue__jki_lib_state_machine.vi"("State(s) in (\"\")"=w713) -> ("States Out"=w712:string)  [unwired: 14 in]
          }
          frame "Macro: Initialize" {
            w714 = "Data: Initialize\nInitialize Core Data\nUI: Initialize\nUI: Front Panel State >> Open"  # Data: Initialize Initialize Core Data UI: Initialize UI: Front Panel State >> Open
            # "Initialization Macro\n(This is called once, when the VI starts)"
            n280 = call <vilib>:"Add State(s) to Queue__jki_lib_state_machine.vi"("State(s) in Front (\"\")"=w714, "State(s) in (\"\")"=w718) -> ("States Out"=w717:string)  [unwired: 13 in]
          }
          frame "Macro: Exit" {
            # "Exit Macro\n(This is called once, when the VI exits)"
            n281 = Unbundle By Name(w725) -> ("Core.Close Panel on Exit?"=w724:bool)
            n282 = Select(t="UI: Front Panel State >> Close", s=w724, f="") -> (s? t:f=w721:string)
            n283 = call <vilib>:"Add State(s) to Queue__jki_lib_state_machine.vi"("State(s) in (\"\")"=w721, "State(s) at Back (\"\")"="Data: Cleanup\nExit") -> ("States Out"=w719:string)  [unwired: 13 in]
            n284 = call <vilib>:"Add State(s) to Queue__jki_lib_state_machine.vi"("State(s) in Front (\"\")"=w719, "State(s) in (\"\")"=w728) -> ("States Out"=w727:string)  [unwired: 13 in]
          }
          frame "---------- New Category ----------" {
            # "Template Separator\n(You can make a copy of, or modify, this frame)"
            n285 = call <vilib>:"Add State(s) to Queue__jki_lib_state_machine.vi"("State(s) in (\"\")"=w732) -> ("States Out"=w731:string)  [unwired: 14 in]
          }
          frame "New Category: 1" {
            # "Your code here.\n(You can make a copy of, or modify, this frame)"
            n286 = control-ref of="2D Picture"() -> (w737:refnum<vi>)
            n287 = Unbundle By Name(w741) -> ("MU Coords"=w740:T4, "MD Coords"=w739:T4)
            n288 = property class="Pict"(reference=w737) -> (reference out=w736:refnum<vi>, "Origin"=w735:T3)  [unwired: 1 in, 1 out]
            n289 = Subtract(x=w740, y=w739) -> (x-y=w738:T4)
            n290 = Negate(x=w738) -> (-x=w734:T4)
            "x-y" <- w734
            n291 = Add(x=w734, y=w735) -> (x+y=w733:T4)
            n292 = property class="Pict"(reference=w736, "Origin"=w733) -> ()  [unwired: 1 in, 2 out]
            n293 = call <vilib>:"Add State(s) to Queue__jki_lib_state_machine.vi"("State(s) in (\"\")"=w744) -> ("States Out"=w743:string)  [unwired: 14 in]
          }
          frame "New Category: 2" {
            # "Your code here.\n(You can make a copy of, or modify, this frame)"
            n294 = call <vilib>:"Add State(s) to Queue__jki_lib_state_machine.vi"("State(s) in (\"\")"=w748) -> ("States Out"=w747:string)  [unwired: 14 in]
          }
        }
      }
      "2D Picture" <- w458
    }
    frame Disabled {
    }
  }
